vi "ScanCtrl_3D.vi"() -> ()   [LabVIEW 2024]
uses:
  <vilib>/Math Plots/3D Math Plots/3D Scatter/3D Scatter XCtrl/3D Scatter.xctl
  <vilib>/userDefined/High Color/IMAQdx.ctl
  <vilib>/vision/Image Controls.llb/IMAQ Image.ctl
  SubVI/GRBL/Status.ctl
  <vilib>/event_ctls.llb/usereventprio.ctl
  <vilib>/vision/driver/IMAQdx.llb/IMAQdx Buffer Number Mode.ctl
  <vilib>/Math Plots/3D Math Plots/3D Scatter/3D Scatter Datatype/Public/Plot Helper (Vector).vi
  <vilib>/Instr/_visa.llb/VISA Configure Serial Port (Instr).vi
  <vilib>/ErrorRing/Error Ring.xnode
  SubVI/GRBL/GRBL 1.1.lvlib
  <userlib>/_OpenG.lib/time/time.llb/openg_time.lvlib
  <vilib>/Math Plots/3D Math Plots/3D Scatter/3D Scatter Datatype/3D Scatter Datatype.lvclass
  <vilib>/vision/driver/NI_Vision_Acquisition_Software.lvlib
panel:
  in  "AbortScan":bool
  out "Estimated surface\n scan time (s)":dbl
  in  "3DProfileScan":bool
  in  "Pre Scan Speed\n(mm/min)":sgl=3000.0
  in  "Y Pixel Size(mm)":dbl=1.0
  in  "Y distance(mm)":dbl=10.0
  in  "X distance (mm)":dbl=10.0
  out "LocationPollingStart":u32
  out "error out":errorcluster
  in  "Save Button":bool
  out "Sys Status":T1
  out "dt polling (ms)":dbl
  out "X encoder count":dbl format="%.2f"
  out "Z Distance(mm)":dbl
  out "X (mm)":dbl
  in  "Range Finder COM":refnum<visa-resource-name>="COM7"
  in  "Stage COM port":refnum<visa-resource-name>="COM6"
  in  "ParseLocationData":bool
  in  "Upper Z limite(mm)":dbl=15.0
  in  "Remove Z outlier":bool
  in  "Probe Radius(2mm)":dbl=2.0 format="%#_13g"
  in  "Interpolate Scan":bool
  in  "FollowScanGridSize(mm)":dbl=0.5 format="%#_13g"
  in  "Calc follow scan":bool
  in  "Follow Z offset(mm)":dbl=3.0
  out "3D Profile":refnum<class "3D Plot Datatype.lvclass">[](xcontrol)
  in  "Follow Speed (mm/min)":sgl=1500.0
  in  "Follow Scan":bool
  in  "Plot 3D":bool
  in  "Tab Control":T2(tab)
  out "Scan Origin MPos":cluster{"X":sgl, "Y":sgl, "Z":sgl}
  in  "Set Origin":bool
  in  "Jog Step Size(mm)":dbl=5.0
  in  "Z--":bool
  in  "Z++":bool
  in  "Y--":bool
  in  "Y++":bool
  in  "X--":bool
  in  "X++":bool
  in  "Hault":bool
  in  "Home":bool
  in  "GoToZero":bool
  out "Current Machine Pos":cluster{"X":sgl, "Y":sgl, "Z":sgl}
  in  "Poll grbl position?":bool
  out "Stage Home MPos":cluster{"X":sgl, "Y":sgl, "Z":sgl}
  in  "Stop":bool
  in  "Start":bool
  in  "AccuRangeLoopStopFlag":bool
  out "read buffer":string
  out "Y Graph":dbl[](graph)
  out "X Graph":dbl[](graph)
  out "Z Graph":dbl[](graph)
  in  "X-Axis configuration":T3={"Travel resolution\t(step/mm)"=160.0, "Maximum rate\t(mm/min)"=6000, "Acceleration\t(mm/sec^2)"=1000, "Maximum travel\t(mm)"=100}
  in  "Y-Axis configuration":T3={"Travel resolution\t(step/mm)"=160.0, "Maximum rate\t(mm/min)"=2000, "Acceleration\t(mm/sec^2)"=250, "Maximum travel\t(mm)"=150}
  in  "Z-Axis configuration":T3={"Travel resolution\t(step/mm)"=160.0, "Maximum rate\t(mm/min)"=2000, "Acceleration\t(mm/sec^2)"=250, "Maximum travel\t(mm)"=70}
  out "Current Config":string="$0=10\r\n$1=255\r\n$2=0\r\n$3=0\r\n$4=0\r\n$5=1\r\n$6=0\r\n$10=1\r\n$11=0.010\r\n$12=1000.000\r\n$13=0\r\n$20=1\r\n$21=0\r\n$22=1\r\n$23=0\r\n$24=5.000\r\n$25=3000.000\r\n$26=25\r\n$27=2.000\r\n$30=12000\r\n$31=4000\r\n$32=0\r\n$100=13.333\r\n$101=13.333\r\n$102=98.000\r\n$110=50000.000\r\n$111=50000.000\r\n$112=1800.000\r\n$120=250.000\r\n$121=250.000\r\n$122=50.000\r\n$130=267.000\r\n$131=472.000\r\n$132=68.000\r\nok\r\nok\r\n"
  out "Version information":string="[VER:1.1f.20170324:]\r\n[OPT:VM,15,128]\r\nok\r\nok\r\n"
  in  "CamSession In":T4="cam0"
  out "New Image":T5
  in  "Preview":bool
  out "Image":T5(plugin-control)
  out "PPIX intensity trace":dbl(graph)
  in  "FollowScan":bool
  out "CH1":refnum<class "3D Plot Datatype.lvclass">[](xcontrol)
  out "AbortFlag":bool
  out "3D scan":errorcluster
  in  "Quit":bool
  # "3D Profile Scan Setting"
  # "Current Position"
  # "Please wait 5s between start and stop"
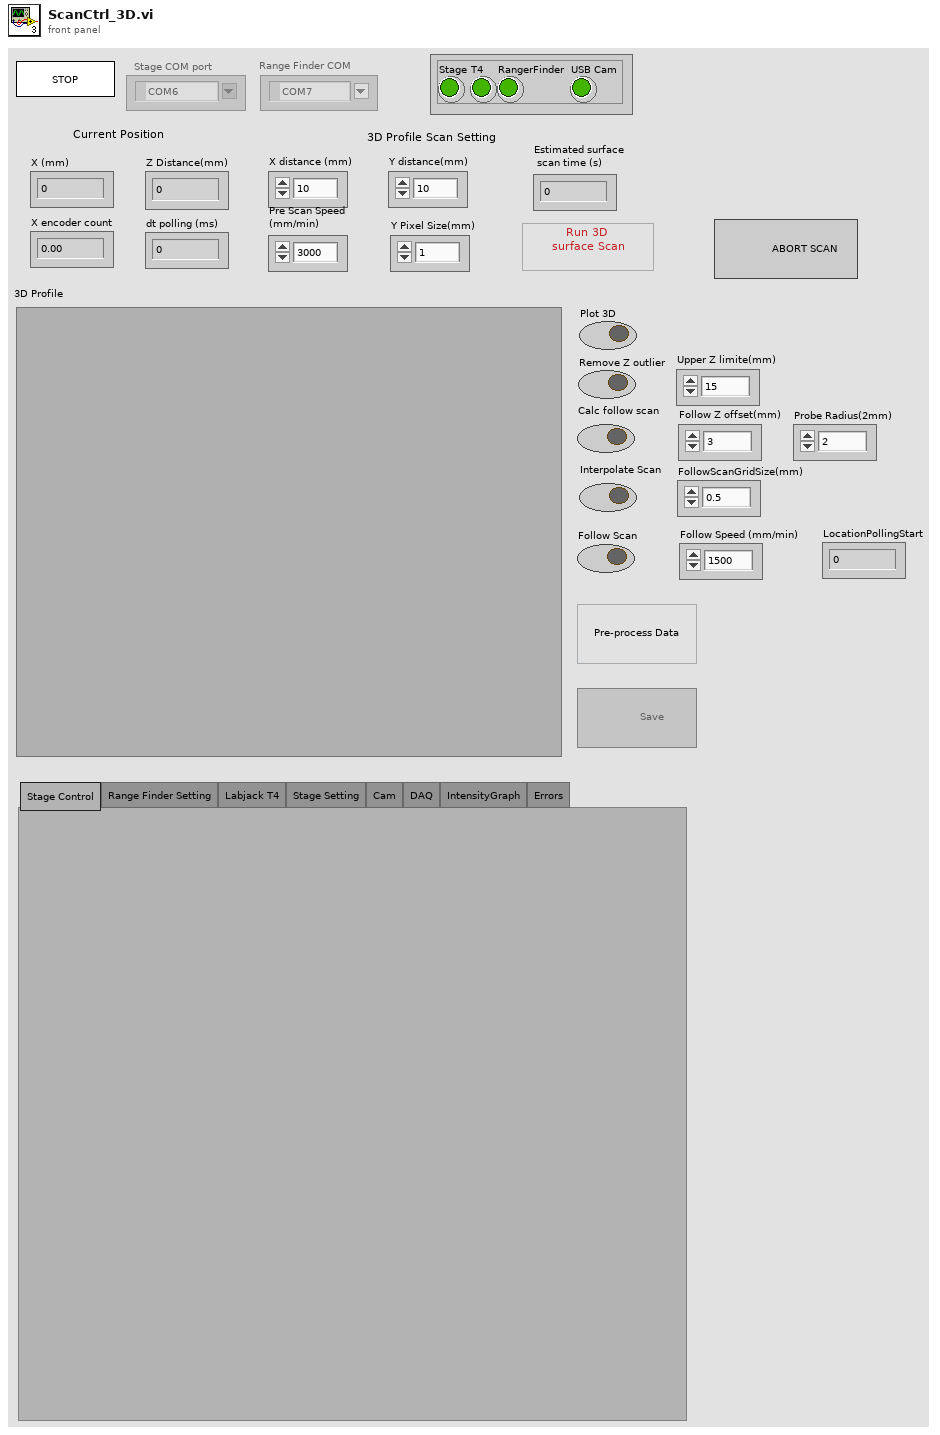
[diagram p1: front panel]
types:
  T1 = cluster{"Stage":bool, "T4":bool, "RangerFinder":bool, "USB Cam":bool}
  T2 = enum32{"Stage Control", "Range Finder Setting", "Labjack T4", "Stage Setting", "Cam", "DAQ", "IntensityGraph", "Errors"}
  T3 = cluster{"Travel resolution\t(step/mm)":sgl, "Maximum rate\t(mm/min)":u32, "Acceleration\t(mm/sec^2)":u32, "Maximum travel\t(mm)":u32}
  T4 = typedef "IMAQdx.ctl" = refnum<k21>
  T5 = typedef "IMAQ Image.ctl" = refnum<image>
  T6 = enum8{"Enabled", "Disabled", "Disabled and Grayed Out"}
  T7 = typedef "NI_Vision_Acquisition_Software.lvlib/IMAQdx Buffer Number Mode.ctl" = enum32{"Next", "Last", "Buffer Number", "Every", "Last New"}
  T8 = typedef "usereventprio.ctl" = enum32{"high priority", "normal priority"}
  T9 = typedef "GRBL 1.1.lvlib/Status.ctl" = enum16{"", "Alarm", "Idle", "Run", "Home"}
  T10 = enum32{"Invalid", "Standard", "Closed", "Hidden", "Minimized", "Maximized"}
  T11 = enum32{"invalid app kind", "Development System", "Run Time System", "Student Edition", "Embedded LabVIEW", "Evaluation", "Custom"}
  T12 = enum16{"open", "open or create", "create or replace", "create", "open (read-only)"}
  T13 = cluster{"Invert enable pin":bool, "Invert limit pin":bool, "Invert probe pin":bool}
  T14 = cluster{"Reverse X":bool, "Reverse Y":bool, "Reverse Z":bool}
  T15 = cluster{"Core":cluster{"Current VI Reference":refnum<vi>, "Close Panel on Exit?":bool}, "Sys Status":cluster{"Stage":bool, "T4":bool, "RangerFinder":bool, "USB Cam":bool}, "StageCOM":refnum<visa-resource-name>, "RangeCOM":refnum<visa-resource-name>, "StepSize":dbl, "ScanOrigin":cluster{"X":sgl, "Y":sgl, "Z":sgl}, "HomeMposOrigin":cluster{"X":sgl, "Y":sgl, "Z":sgl}, "Tic":i32, "IMAQ":T5, "USBCam":T4, "3DProfile":cluster{"x(mm)":dbl, "y(mm)":dbl, "z(mm)":dbl}[], "Raw3DProfile":cluster{"x(mm)":dbl, "y(mm)":dbl, "z(mm)":dbl}[], "FollowScanZOffset(mm)":dbl, "YPixelSize(mm)":dbl, "FollowScanWInter":cluster{"x(mm)":dbl, "y(mm)":dbl, "z(mm)":dbl}[], "BG(V)":dbl, "StageHomed?":bool, "3DProfileToPlot":cluster{"x(mm)":dbl, "y(mm)":dbl, "z(mm)":dbl}[], "FollowScan":cluster{"x(mm)":dbl, "y(mm)":dbl, "z(mm)":dbl}[], "SaveFilePath":path, "Raw3DProfileNoY":cluster{"x(mm)":dbl, "y(mm)":dbl, "z(mm)":dbl}[], "tdms file":refnum<k34>, "FiberOffset":cluster{"x":dbl, "y":dbl}, "RawFollowScanData":cluster{"Time(ms)":dbl, "x":dbl}[], "PPIXProcessedImg":cluster{"x":dbl[], "y":dbl[], "Time(ms)":dbl[]}, "ProbeRadius(mm)":dbl, "FollowGridSize(mm)":dbl}
  T16 = cluster{"remote start event":refnum<user-event>, "remote stop event":refnum<user-event>}
  T17 = cluster{"Current VI Reference":refnum<vi>, "Close Panel on Exit?":bool}
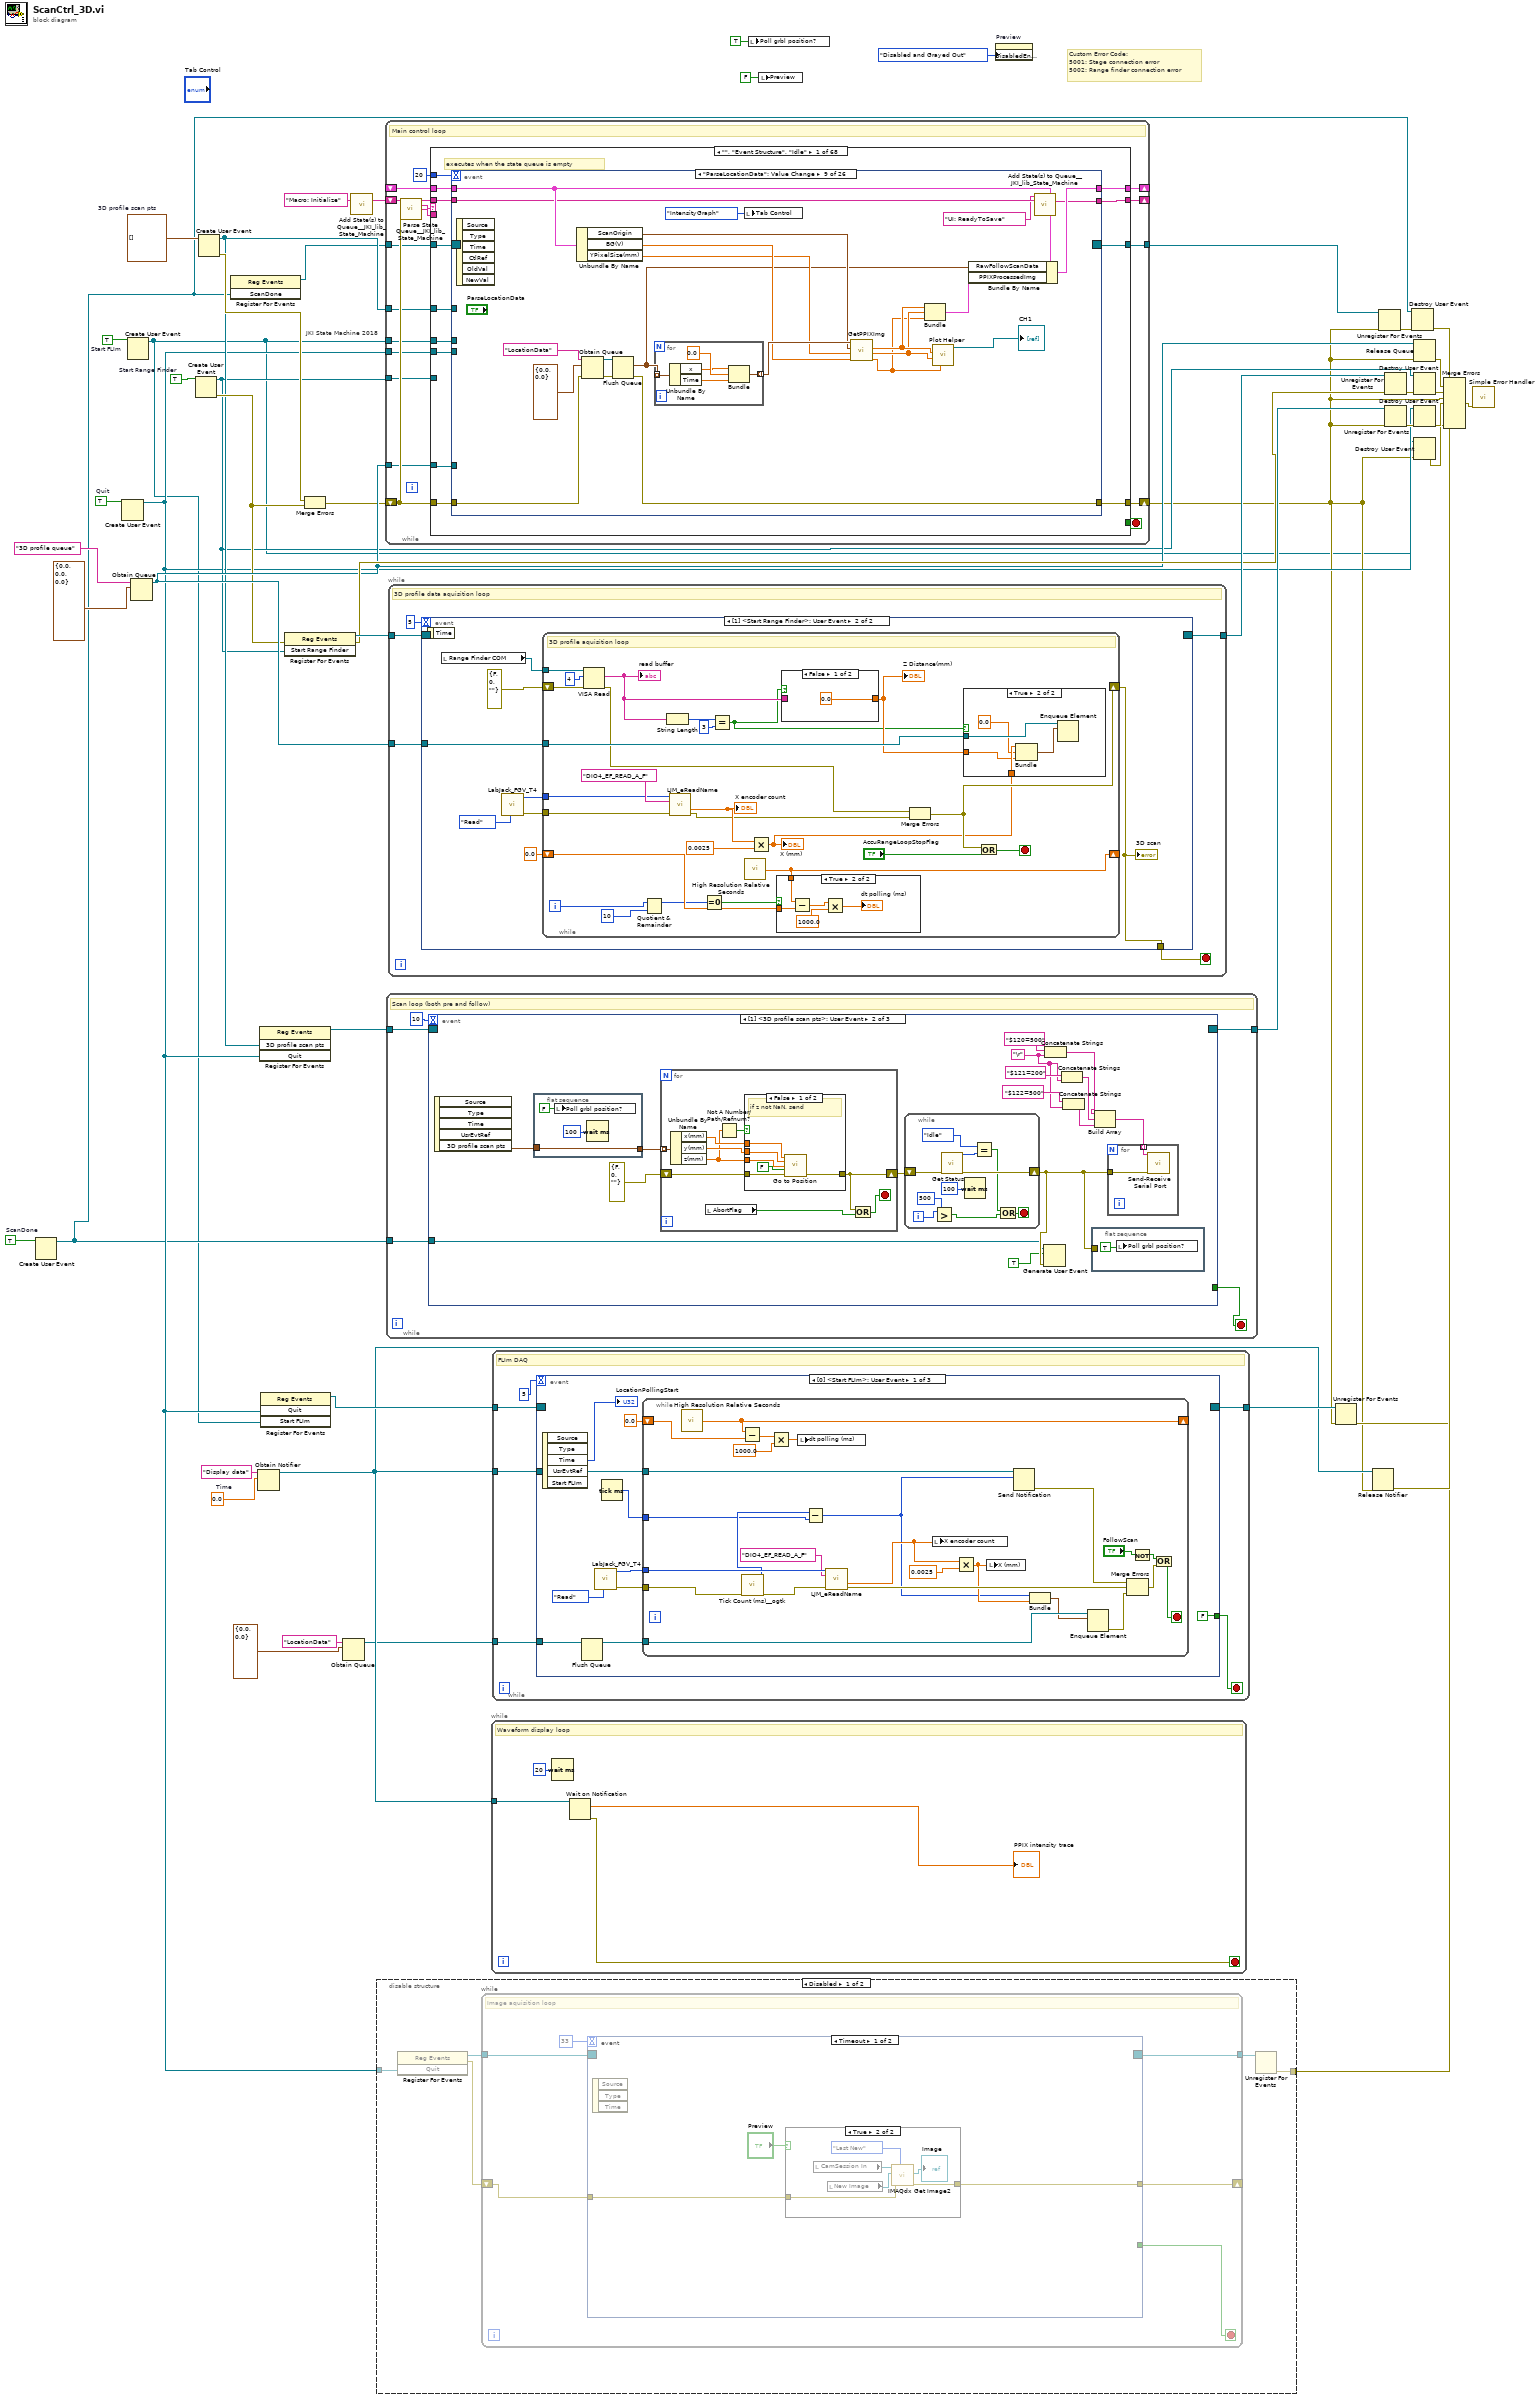
[diagram p0: block diagram]
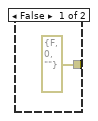
[diagram p2: hidden frame]
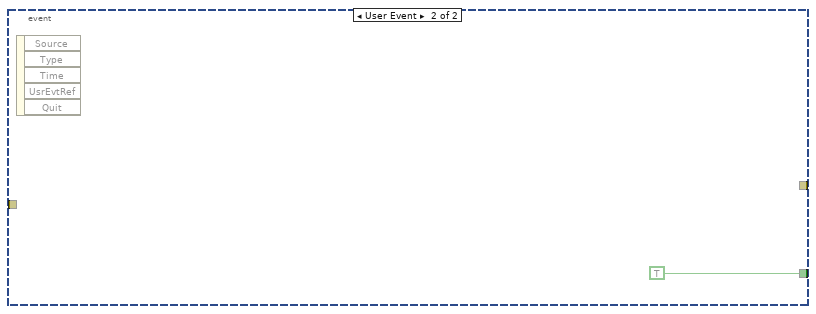
[diagram p3: hidden frame]
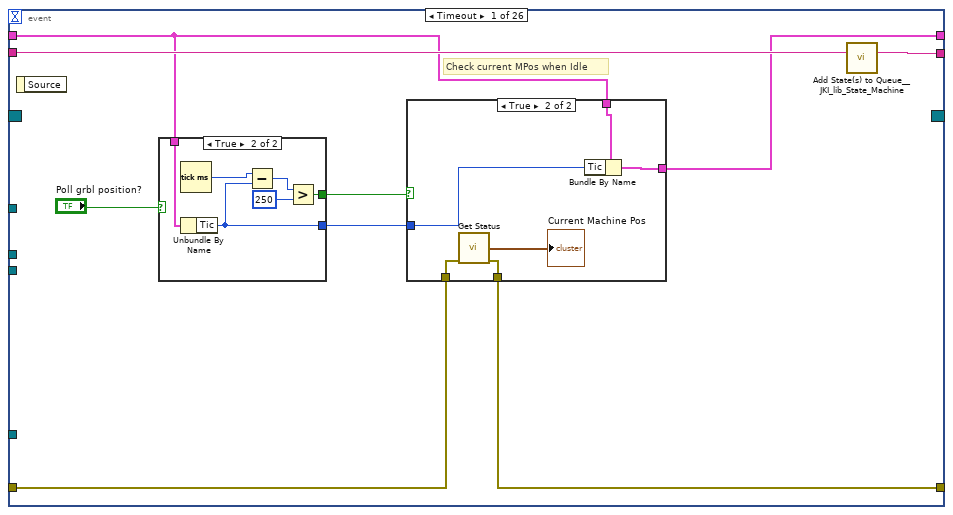
[diagram p5: hidden frame]
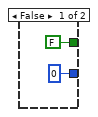
[diagram p6: hidden frame]
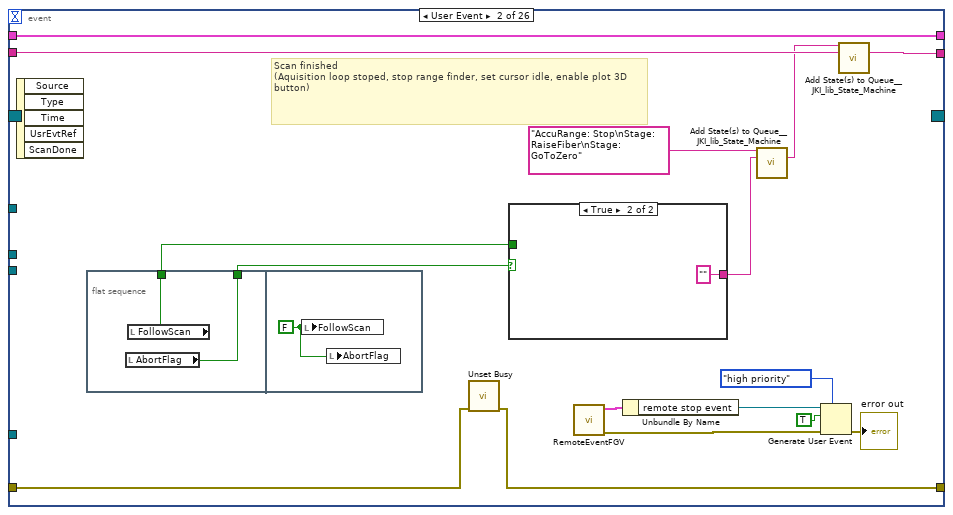
[diagram p8: hidden frame]
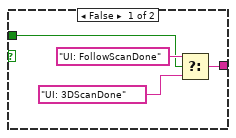
[diagram p9: hidden frame]
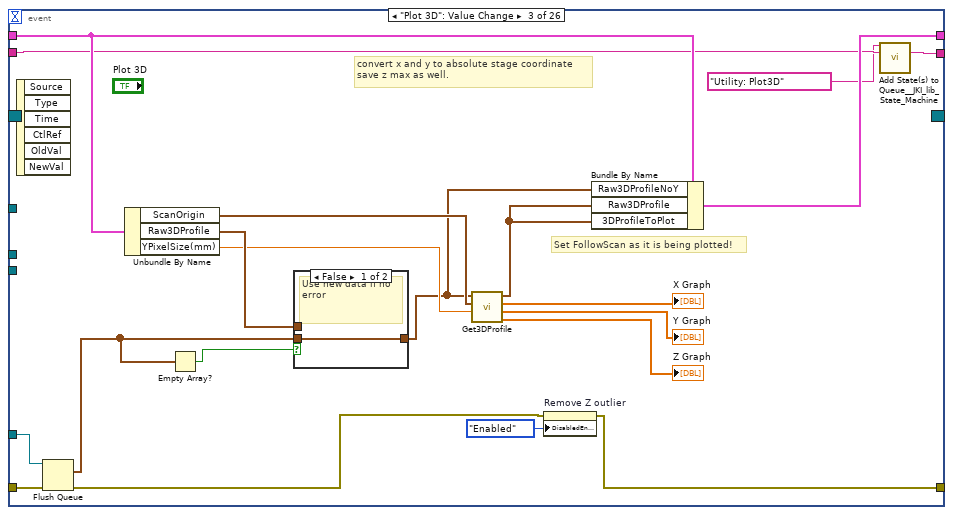
[diagram p10: hidden frame]
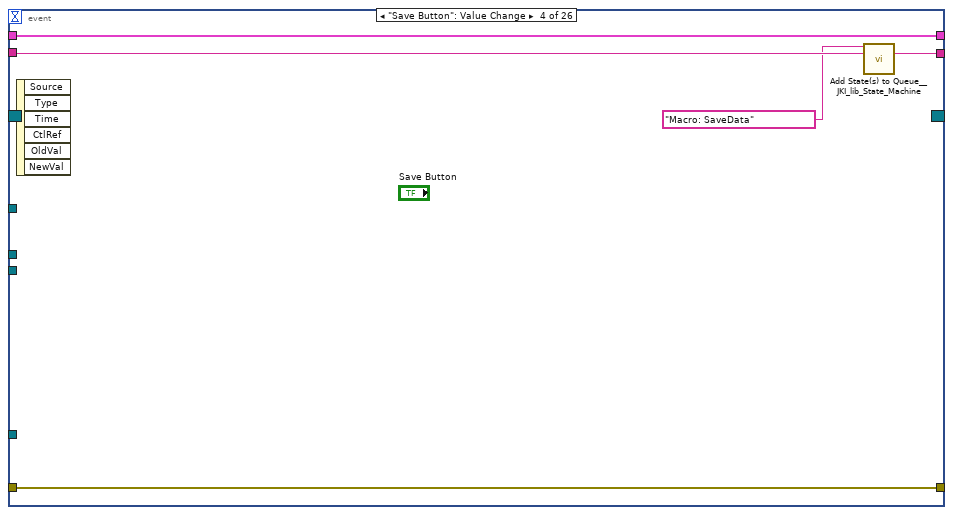
[diagram p12: hidden frame]
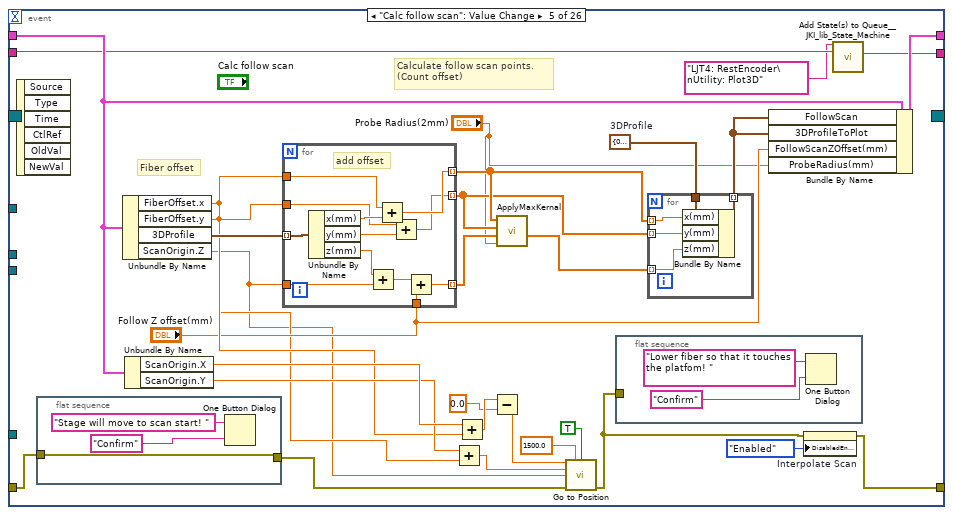
[diagram p13: hidden frame]
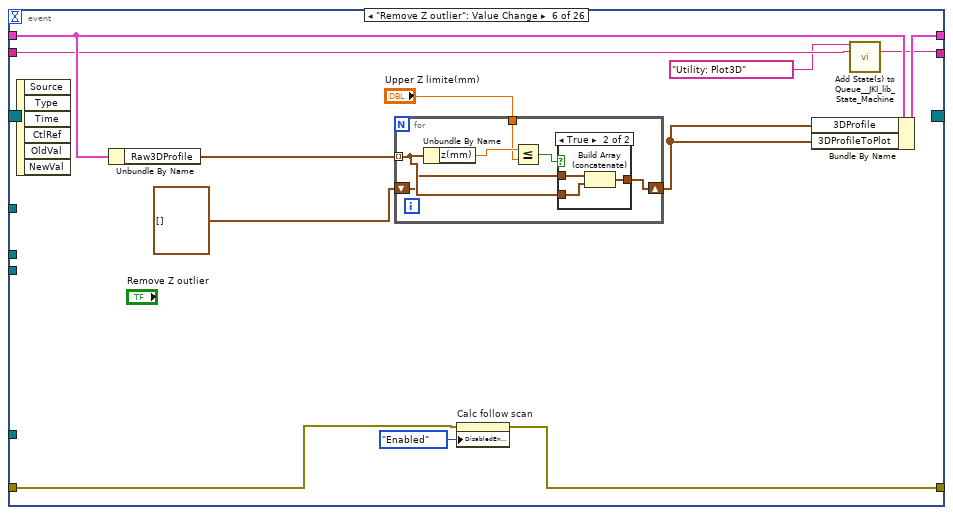
[diagram p14: hidden frame]
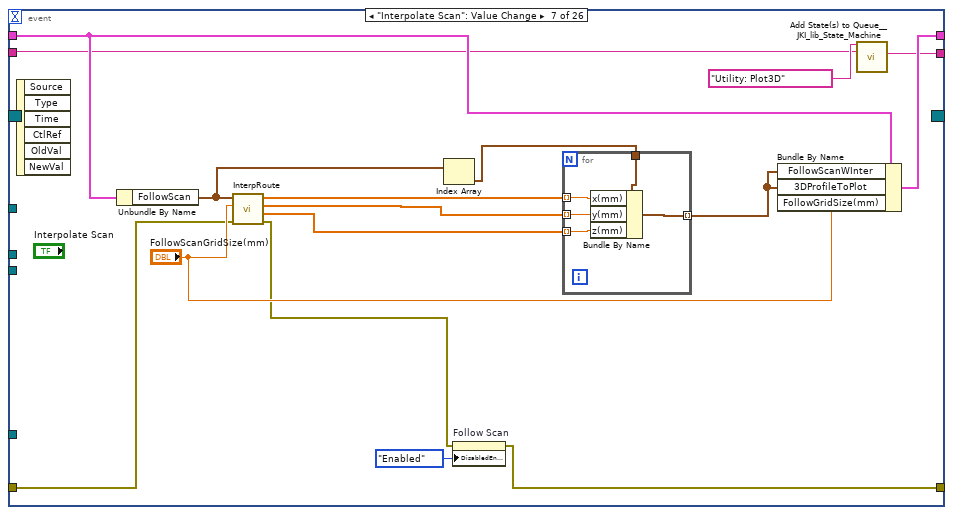
[diagram p16: hidden frame]
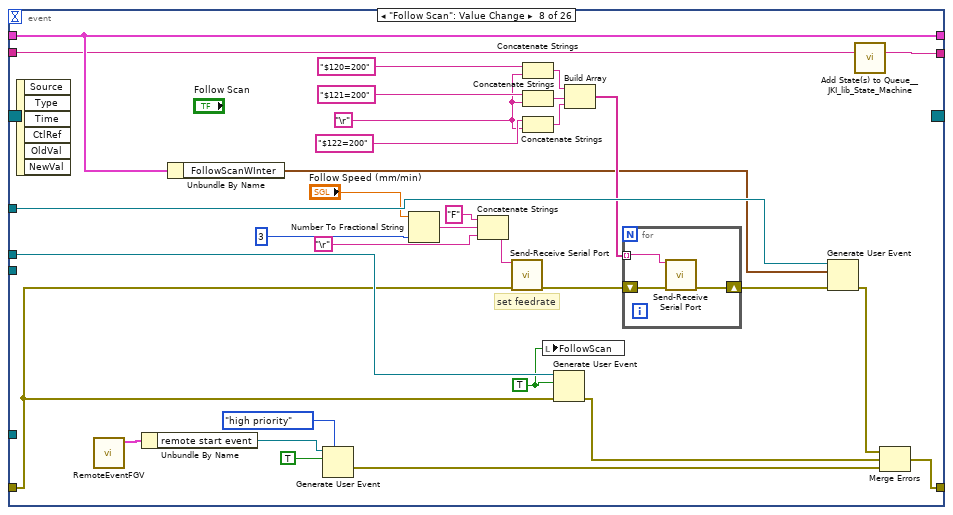
[diagram p17: hidden frame]
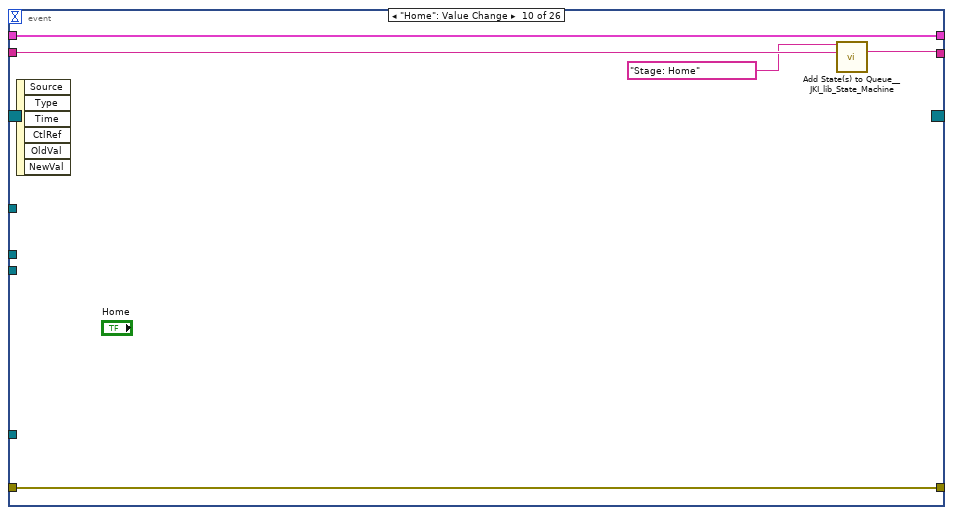
[diagram p18: hidden frame]
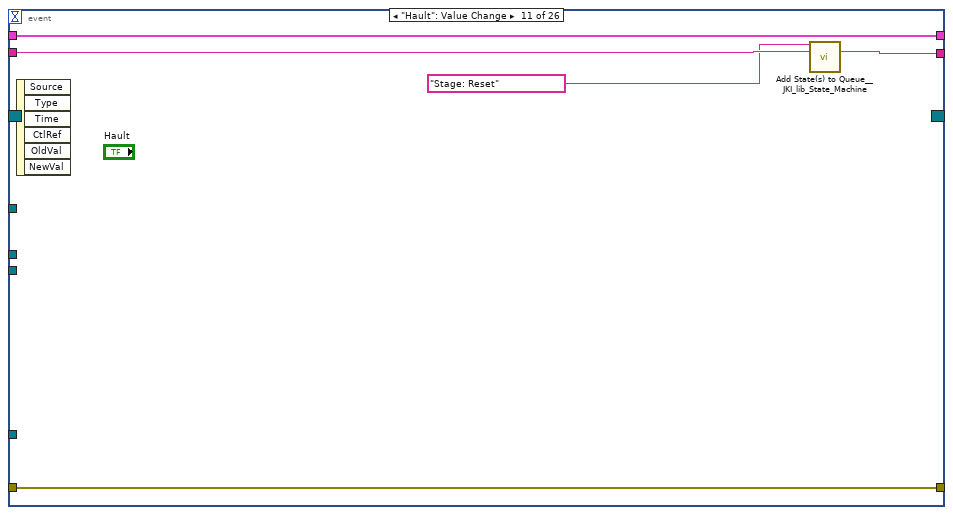
[diagram p19: hidden frame]
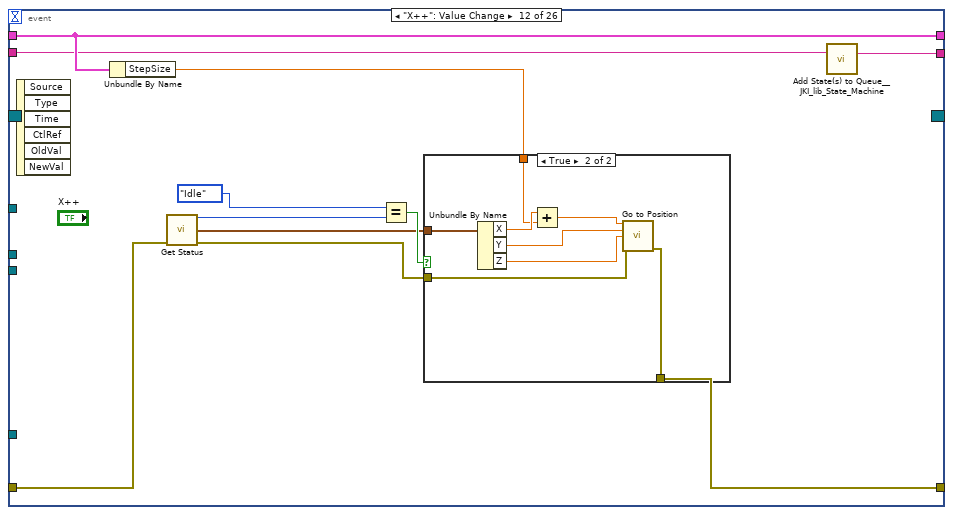
[diagram p20: hidden frame]
diagram:
  w3 = 0.0  # Time
  w12 = TRUE  # ScanDone
  w15 = TRUE  # Start FLIm
  w27 = TRUE  # Quit
  w28 = cluster{"x(mm)":dbl, "y(mm)":dbl, "z(mm)":dbl}[] []  # 3D profile scan pts
  w47 = TRUE  # Start Range Finder
  # "Custom Error Code:\n5001: Stage connection error\n5002: Range finder connection error"
  n1 = Create User Event(user event datatype=w12) -> (user event=w8:refnum<user-event>)  [unwired: 1 in, 1 out]
  n2 = Create User Event(user event datatype=w27) -> (user event=w19:refnum<user-event>)  [unwired: 1 in, 1 out]
  n3 = Create User Event(user event datatype=w15) -> (user event=w1:refnum<user-event>)  [unwired: 1 in, 1 out]
  n4 = Obtain Queue(name (unnamed)="3D profile queue", element data type=cluster{"x(mm)":dbl, "y(mm)":dbl, "z(mm)":dbl} {"x(mm)"=0.0, "y(mm)"=0.0, "z(mm)"=0.0}) -> (queue out=w38:refnum<queue>)  [unwired: 3 in, 2 out]
  n5 = Create User Event(user event datatype=w47) -> (user event=w29:refnum<user-event>, error out=w34:errorcluster)  [unwired: 1 in]
  n6 = Create User Event(user event datatype=w28) -> (user event=w31:refnum<user-event>, error out=w32:errorcluster)  [unwired: 1 in]
  n7 = register-events(w8) -> (reference out=w11:refnum<event-registration>)  [unwired: 2 in, 1 out]
  n8 = Obtain Notifier(name (unnamed)="Display data", notification data type=w3) -> (notifier out=w13:refnum<notifier>)  [unwired: 2 in, 2 out]
  n9 = register-events(w31, w19) -> (reference out=w26:refnum<event-registration>)  [unwired: 2 in, 1 out]
  n10 = register-events(w19, w1) -> (reference out=w22:refnum<event-registration>)  [unwired: 2 in, 1 out]
  n11 = register-events(error in=w34, w29) -> (reference out=w46:refnum<event-registration>, error out=w43:errorcluster)  [unwired: 1 in]
  n12 = Merge Errors(w32, w34) -> (w35:errorcluster)
  n13 = Obtain Queue(name (unnamed)="LocationData", element data type=cluster{"Time":dbl, "x":dbl} {"Time"=0.0, "x"=0.0}) -> (queue out=w4:refnum<queue>)  [unwired: 3 in, 2 out]
  n14 = call <vilib>:"Add State(s) to Queue__JKI_lib_State_Machine.vi"("State(s) in (\"\")"="Macro: Initialize") -> ("States Out"=w49:string)  [unwired: 14 in]
  n15 = disable-structure shown="Disabled" {
    disable-tunnel: w19 -> [w54 _]
    disable-tunnel: [w53 _] -> w18
    frame Disabled {
      n16 = register-events(w54) -> (reference out=w52:refnum<event-registration>, error out=w51:errorcluster)  [unwired: 2 in]
      n17 = while {
        shift-right: [w59] -> _
        shift-left: w51 -> [w58]
        tunnel: w52 -> [w57]
        tunnel: [w55] -> w50
        stop <- w56 stop-if-true
        # "Image aquisition loop"
        n18 = event shown="[0] Timeout" {
          selector: w57 -> [_ _]
          dyn-events: [_ _] -> w55
          timeout: u32 33 ("milliseconds to wait") -> [_ _]
          tunnel: [w62 _] -> w59
          tunnel: w58 -> [w61 _]
          tunnel: [_ TRUE] -> w56
          event Timeout {
            n19 = event-data() -> ()  [unwired: 1 in, 3 out]
            n20 = case shown="True" "Preview" {
              tunnel: [errorcluster {"status"=FALSE, "code"=0, "source"=""} ("error out") w66] -> w62
              tunnel: w61 -> [_ w65]
              frame False {
              }
              frame True {
                n21 = local read "CamSession In"() -> (w68:T4)
                n22 = local read "New Image"() -> (w69:T5)
                n23 = call <vilib>:"IMAQdx Get Image2.vi"("Buffer Number Mode (Next)"=IMAQdx_Buffer_Number_Mode."Last New", "error in"=w65, "Image In"=w69, "Session In"=w68) -> ("error out"=w66:errorcluster, "Image Out"=→"Image":T5)  [unwired: 4 in, 2 out]
              }
            }
          }
          event User Event {
            n24 = event-data() -> ()  [unwired: 1 in, 5 out]
          }
        }
      }
      n25 = Unregister For Events(event registration refnum=w50) -> (error out=w53:errorcluster)  [unwired: 1 in]
    }
    frame Enabled {
    }
  }
  n26 = while "JKI State Machine 2018" {
    shift-right: [w84] -> _
    shift-left: _ -> [w72]
    shift-right: [w87] -> w9
    shift-left: w35 -> [w82]
    shift-right: [w86] -> _
    shift-left: w49 -> [w80]
    tunnel: w29 -> [w81]
    tunnel: w38 -> [w79]
    tunnel: w31 -> [w78]
    tunnel: w19 -> [w77]
    tunnel: w1 -> [w76]
    tunnel: w11 -> [w74]
    tunnel: [w73] -> w10
    stop <- w85 stop-if-true
    # "Main control loop"
    n27 = call <vilib>:"Parse State Queue__JKI_lib_State_Machine.vi"("State Queue"=w80, "Error In (no error)"=w82) -> ("Remaining States"=w89:string, "Current State"=w75:string, "Arguments"=w88:string)  [unwired: 11 in]
    n28 = case shown="\"\", \"Event Structure\", \"Idle\"" w75 {
      selector: w75 -> [_ _ _ _ _ _ w594 _ _ _ _ _ _ _ _ _ _ _ _ _ _ _ _ _ _ _ _ _ _ _ _ _ _ _ _ _ _ _ _ _ _ _ _ _ _ _ _ _ _ _ _ _ _ _ _ _ _ _ _ _ _ _ _ _ _ _ _ _]
      tunnel: w89 -> [w102 w563 w564 w575 w587 w592 w598 w618 w625 w634 w639 w671 w678 w685 w708 w721 w749 w771 w812 w840 w872 w889 w896 w912 w923 w929 w936 w942 w949 w955 w960 w968 w975 w982 w994 w1064 w1076 w1094 w1125 w1136 w1159 w1224 w1244 w1252 w1264 w1280 w1312 w1336 w1349 w1374 w1389 w1399 w1409 w1420 w1425 w1437 w1447 w1465 w1473 w1488 w1505 w1520 w1530 w1545 w1554 w1559 w1564 w1569]
      tunnel: w88 -> [_ _ _ _ _ _ _ _ _ _ _ _ _ _ _ _ _ _ _ _ _ _ _ _ _ _ _ _ _ _ _ _ _ w977 w988 _ _ _ _ _ _ _ w1239 _ _ _ _ _ _ _ _ _ _ w1416 _ _ _ _ _ _ _ _ _ _ _ _ _ _]
      tunnel: w72 -> [w100 w560 w567 w572 w584 w589 w596 w611 w622 w632 w636 _ w674 w680 w702 w718 w746 w768 w809 w837 w869 w886 w893 w903 w920 w926 w933 w939 w946 w952 w957 w965 w973 w980 w990 w1061 w1066 w1092 w1106 w1132 w1153 w1222 w1242 w1246 w1261 w1274 w1310 w1333 w1347 w1367 w1386 w1397 w1405 w1417 w1422 w1432 w1445 w1463 w1467 w1485 w1499 w1513 w1523 w1542 w1550 w1556 w1561 w1566]
      tunnel: [w99 w561 w568 w573 w585 w590 w600 w615 errorcluster {"status"=FALSE, "code"=0, "source"=""} ("error out") w628 w637 w668 w676 w681 w704 w711 w722 w756 w776 w817 w848 w880 w891 w898 w921 w927 w934 w940 w947 w953 w958 w966 w972 w978 w991 w1062 w1070 w1091 w1100 w1134 w1156 w1212 w1241 w1250 w1262 w1265 w1294 w1328 w1343 w1371 w1387 w1392 w1407 w1418 w1423 w1434 w1439 w1450 w1471 w1486 w1498 w1516 w1527 w1543 w1552 w1557 w1562 w1567] -> w87
      tunnel: w82 -> [w98 w561 w568 w573 w585 w590 w599 w615 w621 w627 w637 w668 w676 w682 w703 w716 w729 w755 w797 w825 w862 w882 w890 w897 w921 w927 w934 w940 w947 w953 w958 w966 w972 w979 w992 w1062 w1074 w1090 w1105 w1130 w1157 w1211 w1240 w1249 w1262 w1276 w1295 w1326 w1345 w1370 w1387 w1391 w1407 w1418 w1423 w1430 w1438 w1449 w1470 w1486 w1500 w1515 w1526 w1543 w1552 w1557 w1562 w1567]
      tunnel: [w101 w562 w569 w574 w586 w591 w597 w617 w624 w633 w638 w670 w677 w684 w707 w720 w748 w770 w811 w839 w871 w888 w895 w911 w922 w928 w935 w941 w948 w954 w959 w967 w974 w981 w993 w1063 w1075 w1093 w1124 w1135 w1158 w1223 w1243 w1251 w1263 w1279 w1311 w1335 w1348 w1373 w1388 w1398 w1408 w1419 w1424 w1436 w1446 w1464 w1472 w1487 w1504 w1519 w1529 w1544 w1553 w1558 w1563 w1568] -> w86
      tunnel: [_ _ _ _ _ _ _ _ _ TRUE _ _ _ _ _ _ _ _ _ _ _ _ _ _ _ _ _ _ _ _ _ _ _ _ _ _ _ _ _ _ _ _ _ _ _ _ _ _ _ _ _ _ _ _ _ _ _ _ _ _ _ _ _ _ _ _ _ _] -> w85
      tunnel: [w97 w560 w567 w572 w584 w589 w596 w616 w622 w632 w636 w669 w675 w680 w701 w718 w746 w768 w809 w837 w869 w886 w893 w902 w920 w926 w933 w939 w946 w952 w957 w965 w973 w980 w990 w1061 w1073 w1092 w1106 w1133 w1155 w1222 w1242 w1247 w1261 w1273 w1310 w1333 w1347 w1368 w1386 w1397 w1405 w1417 w1422 w1433 w1445 w1463 w1468 w1485 w1496 w1513 w1524 w1542 w1550 w1556 w1561 w1566] -> w84
      tunnel: 20 ("Timeout") -> [w96 _ _ _ _ _ _ _ _ _ _ _ _ _ _ _ _ _ _ _ _ _ _ _ _ _ _ _ _ _ _ _ _ _ _ _ _ _ _ _ _ _ _ _ _ _ _ _ _ _ _ _ _ _ _ _ _ _ _ _ _ _ _ _ _ _ _ _]
      tunnel: w81 -> [_ _ _ _ _ _ _ _ _ _ _ _ _ _ _ _ _ _ _ _ _ _ _ _ _ _ _ _ _ _ _ _ _ _ _ _ _ _ _ _ _ _ _ _ _ _ _ w1332 _ _ _ _ _ _ _ _ _ _ _ _ _ _ _ _ _ _ _ _]
      tunnel: w79 -> [w95 _ _ _ _ _ _ _ _ _ _ _ _ _ _ _ _ _ _ _ _ _ _ _ _ _ _ _ _ _ _ _ _ _ _ _ _ _ _ _ _ _ _ _ _ _ _ _ _ _ _ _ _ _ _ _ _ _ _ _ _ _ _ _ _ _ _ _]
      tunnel: w78 -> [w94 _ _ _ _ _ _ _ _ _ _ _ _ _ _ _ _ _ _ _ _ _ _ _ _ _ _ _ _ _ _ _ _ _ _ _ _ _ _ _ _ _ _ _ _ _ _ _ _ _ _ _ _ _ _ _ _ _ _ _ _ _ _ _ _ _ _ _]
      tunnel: w77 -> [w93 _ _ _ _ _ _ _ _ w629 _ _ _ _ _ _ _ _ _ _ _ _ _ _ _ _ _ _ _ _ _ _ _ _ _ _ _ _ _ _ _ _ _ _ _ _ _ _ _ _ _ _ _ _ _ _ _ _ _ _ _ _ _ _ _ _ _ _]
      tunnel: w76 -> [w92 _ _ _ _ _ _ _ _ _ _ _ _ _ _ _ _ _ _ _ _ _ _ _ _ _ _ _ _ _ _ _ _ _ _ _ _ _ _ _ _ _ _ _ _ _ _ _ _ _ _ _ _ _ _ _ _ _ _ _ _ _ _ _ _ _ _ _]
      tunnel: w74 -> [w91 w559 w565 w571 w576 w588 w593 w605 w619 w626 w635 w651 w672 w679 w706 w719 w747 w769 w810 w838 w870 w887 w894 w910 w919 w925 w932 w938 w945 w951 w956 w964 w971 w976 w987 w1060 w1068 w1089 w1096 w1131 w1154 w1221 w1238 w1245 w1260 w1266 w1293 w1313 w1339 w1366 w1385 w1396 w1400 w1414 w1421 w1431 w1444 w1448 w1466 w1484 w1489 w1511 w1522 w1541 w1551 w1555 w1560 w1565]
      tunnel: [w90 w559 w565 w571 w576 w588 w593 w605 w619 w626 w635 w651 w672 w679 w706 w719 w747 w769 w810 w838 w870 w887 w894 w910 w919 w925 w932 w938 w945 w951 w956 w964 w971 w976 w987 w1060 w1068 w1089 w1096 w1131 w1154 w1221 w1238 w1245 w1260 w1266 w1293 w1313 w1339 w1366 w1385 w1396 w1400 w1414 w1421 w1431 w1444 w1448 w1466 w1484 w1489 w1511 w1522 w1541 w1551 w1555 w1560 w1565] -> w73
      frame "", "Event Structure", "Idle" {
        # "executes when the state queue is empty"
        n29 = event shown="[8] \"ParseLocationData\": Value Change" {
          selector: w91 -> [_ _ _ _ _ _ _ _ _ _ _ _ _ _ _ _ _ _ _ _ _ _ _ _ _ _]
          dyn-events: [_ _ _ _ _ _ _ _ _ _ _ _ _ _ _ _ _ _ _ _ _ _ _ _ _ _] -> w90
          timeout: w96 -> [_ _ _ _ _ _ _ _ _ _ _ _ _ _ _ _ _ _ _ _ _ _ _ _ _ _]
          tunnel: w102 -> [w111 w141 w165 w176 w197 w238 w259 w285 w311 w338 w344 w354 w375 w389 w401 w422 w443 w463 w478 w508 w520 w535 w542 w546 w551 w558]
          tunnel: [w110 w142 w164 w177 w198 w237 w258 w286 w310 w339 w343 w355 w376 w390 w402 w423 w444 w463 w477 w508 w521 w535 w541 w545 w550 w557] -> w101
          tunnel: w100 -> [w105 w143 w168 w175 w206 w240 w266 w305 w317 w340 w345 w356 w377 w392 w403 w424 w445 w466 w473 w510 w522 w537 w540 w547 w552 w555]
          tunnel: [w109 w131 w154 w178 w200 w233 w261 w281 w325 w337 w341 w347 w368 w391 w394 w415 w436 w456 w470 w511 w513 w533 w538 w543 w548 w556] -> w99
          tunnel: w98 -> [w108 w133 w170 w178 w195 w232 w254 w283 w327 w337 w341 w346 w367 w391 w393 w414 w435 w461 w475 w511 w512 w533 w538 w543 w548 w556]
          tunnel: [w106 w143 w169 w175 w207 w239 w265 w305 w318 w340 w345 w356 w377 w392 w403 w424 w445 w465 w474 w510 w522 w536 w540 w547 w552 w555] -> w97
          tunnel: w95 -> [_ _ w171 _ _ _ _ _ _ _ _ _ _ _ _ _ _ _ w476 _ _ _ _ _ _ _]
          tunnel: w94 -> [_ _ _ _ _ _ _ w304 _ _ _ _ _ _ _ _ _ _ w471 _ _ _ _ _ _ _]
          tunnel: w93 -> [_ _ _ _ _ _ _ _ _ _ _ _ _ _ _ _ _ _ _ _ _ _ _ _ _ _]
          tunnel: w92 -> [_ _ _ _ _ _ _ w284 _ _ _ _ _ _ _ _ _ _ _ _ _ _ _ _ _ _]
          event Timeout {
            # "Check current MPos when Idle"
            n30 = event-data() -> ()  [unwired: 1 in, 1 out]
            n31 = case shown="True" "Poll grbl position?" {
              tunnel: [FALSE w116] -> w107
              tunnel: w105 -> [_ w115]
              tunnel: [0 ("Tic") w114] -> w104
              frame False {
              }
              frame True {
                n32 = Tick Count (ms)() -> (millisecond timer value=w119:u32)
                n33 = Unbundle By Name(w115) -> ("Tic"=w114:i32)
                n34 = Subtract(x=w119, y=w114) -> (x-y=w118:u32)
                n35 = Greater?(x=w118, y=u32 250) -> (0:w116:bool)
              }
            }
            n36 = case shown="True" w107 {
              tunnel: [w121 w127] -> w109
              tunnel: w108 -> [w121 w126]
              tunnel: w105 -> [w120 w124]
              tunnel: [w120 w123] -> w106
              tunnel: w104 -> [_ w122]
              frame False {
              }
              frame True {
                n37 = call "Get Status.vi"("error in (no error)"=w126) -> ("Current position"=→"Current Machine Pos":cluster{"X":sgl, "Y":sgl, "Z":sgl}, "error out"=w127:errorcluster)  [unwired: 10 in, 3 out]
                n38 = Bundle By Name(cluster=w124, "Tic"=w122) -> (w123:T15)
              }
            }
            n39 = call <vilib>:"Add State(s) to Queue__JKI_lib_State_Machine.vi"("State(s) in (\"\")"=w111) -> ("States Out"=w110:string)  [unwired: 14 in]
          }
          event User Event {
            # "Scan finished\n(Aquisition loop stoped, stop range finder, set cursor idle, enable plot 3D button)"
            n40 = event-data() -> ()  [unwired: 1 in, 5 out]
            n41 = flat-sequence {
              tunnel: [w150] -> w140
              tunnel: [w149] -> w128
              frame #0 {
                n42 = local read "AbortFlag"() -> (w149:bool)
                n43 = local read "FollowScan"() -> (w150:bool)
              }
              frame #1 {
                w151 = FALSE ("InScan")
                n44 = local write "FollowScan"(w151) -> ()
                n45 = local write "AbortFlag"(w151) -> ()
              }
            }
            n46 = call <vilib>:"Unset Busy.vi"("error in (no error)"=w133) -> ("error out"=w131:errorcluster)  [unwired: 10 in]
            n47 = case shown="True" w128 {
              tunnel: w140 -> [w145 _]
              tunnel: [w144 "" ("State(s) in (\"\")")] -> w138
              frame False {
                n48 = Select(t="UI: FollowScanDone", s=w145, f="UI: 3DScanDone" ("State(s) in (\"\")")) -> (s? t:f=w144:string)
              }
              frame True {
              }
            }
            n49 = call "RemoteEventFGV.vi"() -> ("Error Out"=w132:errorcluster, "Remote Event out"=w136:T16)  [unwired: 10 in]
            n50 = Unbundle By Name(w136) -> ("remote stop event"=w135:refnum<user-event>)
            n51 = call <vilib>:"Add State(s) to Queue__JKI_lib_State_Machine.vi"("State(s) in Front (\"\")"="AccuRange: Stop\nStage: RaiseFiber\nStage: GoToZero" ("State(s) in (\"\")"), "State(s) in (\"\")"=w138) -> ("States Out"=w137:string)  [unwired: 13 in]
            n52 = Generate User Event(priority (normal)=usereventprio."high priority", user event=w135, event data cluster=TRUE ("event data"), error in=w132) -> (error out=→"error out":errorcluster)  [unwired: 1 out]
            n53 = call <vilib>:"Add State(s) to Queue__JKI_lib_State_Machine.vi"("State(s) in Front (\"\")"=w137, "State(s) in (\"\")"=w141) -> ("States Out"=w142:string)  [unwired: 13 in]
          }
          event "Plot 3D": Value Change {
            # "Set FollowScan as it is being plotted!"
            # "convert x and y to absolute stage coordinate\nsave z max as well."
            n54 = event-data() -> ()  [unwired: 1 in, 6 out]
            n55 = Flush Queue(queue=w171, error in (no error)=w170) -> (remaining elements=w159:cluster{"x(mm)":dbl, "y(mm)":dbl, "z(mm)":dbl}[], error out=w155:errorcluster)  [unwired: 1 out]
            n56 = Unbundle By Name(w168) -> ("ScanOrigin"=w167:cluster{"X":sgl, "Y":sgl, "Z":sgl}, "Raw3DProfile"=w162:cluster{"x(mm)":dbl, "y(mm)":dbl, "z(mm)":dbl}[], "YPixelSize(mm)"=w161:dbl)
            n57 = Empty Array?(array=w159) -> (empty?=w158:bool)
            n58 = case shown="False" w158 {
              tunnel: w159 -> [w172 _]
              tunnel: [w172 w173] -> w152
              tunnel: w162 -> [_ w173]
              frame False {
                # "Use new data if no error"
              }
              frame True {
                # "Use old data if error"
              }
            }
            n59 = call "Get3DProfile.vi"("dy"=w161, "Origin"=w167, "remaining elements"=w152) -> ("Z"=→"Z Graph":dbl[], "Y"=→"Y Graph":dbl[], "X"=→"X Graph":dbl[], "3D Profile"=w156:cluster{"x(mm)":dbl, "y(mm)":dbl, "z(mm)":dbl}[])  [unwired: 5 in]
            n60 = property on="Remove Z outlier" class="Bool"(error in=w155, "DisabledEnum"=T6."Enabled" ("Disabled")) -> (error out=w154:errorcluster)  [unwired: 1 in, 1 out]
            n61 = Bundle By Name(cluster=w168, "Raw3DProfileNoY"=w152, "Raw3DProfile"=w156, "3DProfileToPlot"=w156) -> (w169:T15)
            n62 = call <vilib>:"Add State(s) to Queue__JKI_lib_State_Machine.vi"("State(s) in Front (\"\")"="Utility: Plot3D" ("State(s) in Front (\"\")"), "State(s) in (\"\")"=w165) -> ("States Out"=w164:string)  [unwired: 13 in]
          }
          event "Save Button": Value Change {
            n63 = event-data() -> ()  [unwired: 1 in, 6 out]
            n64 = call <vilib>:"Add State(s) to Queue__JKI_lib_State_Machine.vi"("State(s) in Front (\"\")"="Macro: SaveData" ("State(s) in Front (\"\")"), "State(s) in (\"\")"=w176) -> ("States Out"=w177:string)  [unwired: 13 in]
          }
          event "Calc follow scan": Value Change {
            w188 = cluster{"x(mm)":dbl, "y(mm)":dbl, "z(mm)":dbl} {"x(mm)"=0.0, "y(mm)"=0.0, "z(mm)"=0.0}  # 3DProfile
            # "Fiber offset"
            # "Calculate follow scan points.\n(Count offset)"
            n65 = event-data() -> ()  [unwired: 1 in, 6 out]
            n66 = flat-sequence {
              tunnel: w195 -> [w216]
              tunnel: [w216] -> w179
              frame #0 {
                n67 = One Button Dialog(message="Stage will move to scan start! ", button name ("OK")="Confirm") -> ()  [unwired: 1 out]
              }
            }
            n68 = Unbundle By Name(w206) -> ("FiberOffset.x"=w193:dbl, "FiberOffset.y"=w185:dbl, "3DProfile"=w208:cluster{"x(mm)":dbl, "y(mm)":dbl, "z(mm)":dbl}[], "ScanOrigin.Z"=w184:sgl)
            n69 = Unbundle By Name(w206) -> ("ScanOrigin.X"=w205:sgl, "ScanOrigin.Y"=w201:sgl)
            n70 = for {
              tunnel: w208 -> [w230] mode=indexing
              tunnel: w184 -> [w229]
              tunnel: "Follow Z offset(mm)" -> [w227]
              tunnel: w193 -> [w223]
              tunnel: w185 -> [w222]
              tunnel: [w221] -> w189 mode=indexing
              tunnel: [w220] -> w187 mode=indexing
              tunnel: [w219] -> w191 mode=indexing
              # "add offset"
              n71 = Unbundle By Name(w230) -> ("x(mm)"=w226:dbl, "y(mm)"=w225:dbl, "z(mm)"=w224:dbl)
              n72 = Add(x=w224, y=w229) -> (x+y=w228:dbl)
              n73 = Add(x=w223, y=w226) -> (x+y=w221:dbl)
              n74 = Add(x=w222, y=w225) -> (x+y=w220:dbl)
              n75 = Add(x=w228, y=w227) -> (x+y=w219:dbl)
            }
            n76 = Add(x=w201, y=w185) -> (x+y=w204:dbl)
            n77 = Add(x=w205, y=w193) -> (x+y=w182:dbl)
            n78 = Subtract(x=w182, y=0.0) -> (x-y=w180:dbl)
            n79 = call "ApplyMaxKernal.vi"("Radius(2mm)"="Probe Radius(2mm)", "Z"=w191, "Y"=w187, "X"=w189) -> ("ZZ"=w190:dbl[])  [unwired: 7 in]
            n80 = call "Go to Position.vi"("X (mm)"=w180, "Speed (2000 mm/min)"=sgl 1500.0 ("Speed (mm/min)"), "Overwright speed? (F)"=TRUE, "Y (mm)"=w204, "Z (mm)"=w184, "error in (no error)"=w179) -> ("error out"=w194:errorcluster)  [unwired: 9 in]
            n81 = flat-sequence {
              tunnel: w194 -> [_]
              frame #0 {
                n82 = One Button Dialog(message="Lower fiber so that it touches the platfom! ", button name ("OK")="Confirm") -> ()  [unwired: 1 out]
              }
            }
            n83 = for {
              tunnel: w190 -> [w210] mode=indexing
              tunnel: w189 -> [w212] mode=indexing
              tunnel: w188 -> [w213]
              tunnel: w187 -> [w211] mode=indexing
              tunnel: [w209] -> w186 mode=indexing
              n84 = Bundle By Name(cluster=w213, "x(mm)"=w212, "y(mm)"=w211, "z(mm)"=w210) -> (w209:cluster{"x(mm)":dbl, "y(mm)":dbl, "z(mm)":dbl})
            }
            n85 = Bundle By Name(cluster=w206, "FollowScan"=w186, "3DProfileToPlot"=w186, "FollowScanZOffset(mm)"="Follow Z offset(mm)", "ProbeRadius(mm)"="Probe Radius(2mm)") -> (w207:T15)
            n86 = property on="Interpolate Scan" class="Bool"(error in=w194, "DisabledEnum"=T6."Enabled" ("Disabled")) -> (error out=w200:errorcluster)  [unwired: 1 in, 1 out]
            n87 = call <vilib>:"Add State(s) to Queue__JKI_lib_State_Machine.vi"("State(s) in Front (\"\")"="LJT4: RestEncoder\nUtility: Plot3D" ("State(s) in Front (\"\")"), "State(s) in (\"\")"=w197) -> ("States Out"=w198:string)  [unwired: 13 in]
          }
          event "Remove Z outlier": Value Change {
            n88 = event-data() -> ()  [unwired: 1 in, 6 out]
            n89 = Unbundle By Name(w240) -> ("Raw3DProfile"=w241:cluster{"x(mm)":dbl, "y(mm)":dbl, "z(mm)":dbl}[])
            n90 = for {
              tunnel: w241 -> [w244] mode=indexing
              tunnel: "Upper Z limite(mm)" -> [w247]
              shift-right: [w245] -> w231
              shift-left: cluster{"x(mm)":dbl, "y(mm)":dbl, "z(mm)":dbl}[] [] -> [w243]
              n91 = Unbundle By Name(w244) -> ("z(mm)"=w248:dbl)
              n92 = Less Or Equal?(x=w248, y=w247) -> (x <= y?=w246:bool)
              n93 = case shown="True" w246 {
                tunnel: [w249 w252] -> w245
                tunnel: w244 -> [_ w251]
                tunnel: w243 -> [w249 w250]
                frame False {
                }
                frame True {
                  n94 = Build Array (concatenate)(w250, w251) -> (w252:cluster{"x(mm)":dbl, "y(mm)":dbl, "z(mm)":dbl}[])
                }
              }
            }
            n95 = property on="Calc follow scan" class="Bool"(error in=w232, "DisabledEnum"=T6."Enabled" ("Disabled")) -> (error out=w233:errorcluster)  [unwired: 1 in, 1 out]
            n96 = Bundle By Name(cluster=w240, "3DProfile"=w231, "3DProfileToPlot"=w231) -> (w239:T15)
            n97 = call <vilib>:"Add State(s) to Queue__JKI_lib_State_Machine.vi"("State(s) in Front (\"\")"="Utility: Plot3D" ("State(s) in Front (\"\")"), "State(s) in (\"\")"=w238) -> ("States Out"=w237:string)  [unwired: 13 in]
          }
          event "Interpolate Scan": Value Change {
            n98 = event-data() -> ()  [unwired: 1 in, 6 out]
            n99 = Unbundle By Name(w266) -> ("FollowScan"=w268:cluster{"x(mm)":dbl, "y(mm)":dbl, "z(mm)":dbl}[])
            n100 = call "InterpRoute.vi"("error in (no error)"=w254, "GridSize(mm)"="FollowScanGridSize(mm)", "FollowScanWOffset"=w268) -> ("error out"=w253:errorcluster, "Zi"=w256:dbl[], "Yi"=w263:dbl[], "Xi"=w264:dbl[])  [unwired: 4 in, 1 out]
            n101 = Index Array(array=w268) -> (element=w267:cluster{"x(mm)":dbl, "y(mm)":dbl, "z(mm)":dbl})  [unwired: 1 in]
            n102 = property on="Follow Scan" class="Bool"(error in=w253, "DisabledEnum"=T6."Enabled" ("Disabled")) -> (error out=w261:errorcluster)  [unwired: 1 in, 1 out]
            n103 = for {
              tunnel: w267 -> [w273]
              tunnel: w264 -> [w272] mode=indexing
              tunnel: w263 -> [w271] mode=indexing
              tunnel: w256 -> [w270] mode=indexing
              tunnel: [w269] -> w257 mode=indexing
              n104 = Bundle By Name(cluster=w273, "x(mm)"=w272, "y(mm)"=w271, "z(mm)"=w270) -> (w269:cluster{"x(mm)":dbl, "y(mm)":dbl, "z(mm)":dbl})
            }
            n105 = Bundle By Name(cluster=w266, "FollowScanWInter"=w257, "3DProfileToPlot"=w257, "FollowGridSize(mm)"="FollowScanGridSize(mm)") -> (w265:T15)
            n106 = call <vilib>:"Add State(s) to Queue__JKI_lib_State_Machine.vi"("State(s) in Front (\"\")"="Utility: Plot3D" ("State(s) in Front (\"\")"), "State(s) in (\"\")"=w259) -> ("States Out"=w258:string)  [unwired: 13 in]
          }
          event "Follow Scan": Value Change {
            w280 = TRUE ("event data")
            w292 = "\r"
            # "set feedrate"
            n107 = event-data() -> ()  [unwired: 1 in, 6 out]
            n108 = call "RemoteEventFGV.vi"() -> ("Remote Event out"=w278:T16)  [unwired: 10 in, 1 out]
            n109 = Unbundle By Name(w278) -> ("remote start event"=w277:refnum<user-event>)
            n110 = Unbundle By Name(w305) -> ("FollowScanWInter"=w287:cluster{"x(mm)":dbl, "y(mm)":dbl, "z(mm)":dbl}[])
            n111 = Generate User Event(priority (normal)=usereventprio."high priority", user event=w277, event data cluster=TRUE ("event data")) -> (error out=w274:errorcluster)  [unwired: 1 in, 1 out]
            n112 = Number To Fractional String(number="Follow Speed (mm/min)", precision (6)=i16 3) -> (F-format string=w301:string)  [unwired: 2 in]
            n113 = Concatenate Strings("F" ("string"), w301, "\r") -> (w300:string)
            n114 = call "Send-Receive Serial Port.vi"("Data to write"=w300, "error in (no error)"=w283) -> ("error out"=w297:errorcluster)  [unwired: 12 in, 1 out]
            n115 = Concatenate Strings("$120=200" ("string"), w292) -> (w291:string)
            n116 = Concatenate Strings("$121=200" ("string"), w292) -> (w290:string)
            n117 = Concatenate Strings("$122=200" ("string"), w292) -> (w289:string)
            n118 = local write "FollowScan"(w280) -> ()
            n119 = Generate User Event(user event=w284, event data cluster=w280, error in=w283) -> (error out=w279:errorcluster)  [unwired: 1 in, 1 out]
            n120 = Build Array(w291, w290, w289) -> (w288:string[])
            n121 = for {
              shift-right: [w307] -> w296
              shift-left: w297 -> [w308]
              tunnel: w288 -> [w306] mode=indexing
              n122 = call "Send-Receive Serial Port.vi"("Data to write"=w306, "error in (no error)"=w308) -> ("error out"=w307:errorcluster)  [unwired: 12 in, 1 out]
            }
            n123 = Generate User Event(user event=w304, event data cluster=w287, error in=w296) -> (error out=w282:errorcluster)  [unwired: 1 in, 1 out]
            n124 = call <vilib>:"Add State(s) to Queue__JKI_lib_State_Machine.vi"("State(s) in (\"\")"=w285) -> ("States Out"=w286:string)  [unwired: 14 in]
            n125 = Merge Errors(w282, w279, w274) -> (w281:errorcluster)
          }
          event "ParseLocationData": Value Change {
            n126 = event-data() -> ()  [unwired: 1 in, 6 out]
            n127 = Unbundle By Name(w317) -> ("ScanOrigin"=w322:cluster{"X":sgl, "Y":sgl, "Z":sgl}, "BG(V)"=w321:dbl, "YPixelSize(mm)"=w319:dbl)
            n128 = Obtain Queue(name (unnamed)="LocationData", element data type=cluster{"Time":dbl, "x":dbl} {"Time"=0.0, "x"=0.0}, error in (no error)=w327) -> (queue out=w328:refnum<queue>, error out=w329:errorcluster)  [unwired: 2 in, 1 out]
            n129 = Flush Queue(queue=w328, error in (no error)=w329) -> (remaining elements=w316:cluster{"Time":dbl, "x":dbl}[], error out=w325:errorcluster)  [unwired: 1 out]
            n130 = for {
              tunnel: w316 -> [w335] mode=indexing
              tunnel: [w333] -> w323 mode=indexing
              n131 = Unbundle By Name(w335) -> ("x"=w332:dbl, "Time"=w331:dbl)
              n132 = Bundle("x"=w332, 0.0, "Time"=w331) -> (w333:cluster{"x":dbl, dbl, "Time":dbl})  [unwired: 1 in]
            }
            n133 = local write "Tab Control"(T2."IntensityGraph" ("Tab Control")) -> ()
            n134 = call "GetPPIXImg.vi"("Background"=w321, "dy"=w319, "Origin"=w322, "3D Profile in"=w323) -> ("Z"=w313:dbl[], "Y"=w314:dbl[], "X"=w315:dbl[])  [unwired: 4 in, 1 out]
            n135 = Bundle("X"=w315, "Y"=w314, "Z"=w313) -> (w312:cluster{"X":dbl[], "Y":dbl[], "Z":dbl[]})  [unwired: 1 in]
            n136 = call-poly <vilib>:"Plot Helper.vi"("z vector"=w313, "y vector"=w314, "x vector"=w315) -> ("3D Plot lvclass Array out"=→"CH1":refnum<class "3D Plot Datatype.lvclass">[])  [unwired: 3 in, 5 out]
            n137 = Bundle By Name(cluster=w317, "RawFollowScanData"=w316, "PPIXProcessedImg"=w312) -> (w318:T15)
            n138 = call <vilib>:"Add State(s) to Queue__JKI_lib_State_Machine.vi"("State(s) in Front (\"\")"="UI: ReadyToSave" ("State(s) in Front (\"\")"), "State(s) in (\"\")"=w311) -> ("States Out"=w310:string)  [unwired: 13 in]
          }
          event "Home": Value Change {
            n139 = event-data() -> ()  [unwired: 1 in, 6 out]
            n140 = call <vilib>:"Add State(s) to Queue__JKI_lib_State_Machine.vi"("State(s) in Front (\"\")"="Stage: Home" ("State(s) in Front (\"\")"), "State(s) in (\"\")"=w338) -> ("States Out"=w339:string)  [unwired: 13 in]
          }
          event "Hault": Value Change {
            n141 = event-data() -> ()  [unwired: 1 in, 6 out]
            n142 = call <vilib>:"Add State(s) to Queue__JKI_lib_State_Machine.vi"("State(s) in Front (\"\")"="Stage: Reset" ("State(s) in Front (\"\")"), "State(s) in (\"\")"=w344) -> ("States Out"=w343:string)  [unwired: 13 in]
          }
          event "X++": Value Change {
            n143 = event-data() -> ()  [unwired: 1 in, 6 out]
            n144 = Unbundle By Name(w356) -> ("StepSize"=w349:dbl)
            n145 = call "Get Status.vi"("error in (no error)"=w346) -> ("Status"=w353:T9, "Current position"=w350:cluster{"X":sgl, "Y":sgl, "Z":sgl}, "error out"=w348:errorcluster)  [unwired: 10 in, 2 out]
            n146 = Equal?(x=Status."Idle" ("Status"), y=w353) -> (x = y?=w351:bool)
            n147 = case shown="True" w351 {
              tunnel: w350 -> [_ w366]
              tunnel: w349 -> [_ w359]
              tunnel: w348 -> [w358 w362]
              tunnel: [w358 w361] -> w347
              frame False {
                n148 = One Button Dialog(message="Stage is not Idle!\nPlease try again when stage is Idle. ") -> ()  [unwired: 1 in, 1 out]
              }
              frame True {
                n149 = Unbundle By Name(w366) -> ("X"=w360:sgl, "Y"=w364:sgl, "Z"=w363:sgl)
                n150 = Add(x=w360, y=w359) -> (x+y=w365:dbl)
                n151 = call "Go to Position.vi"("X (mm)"=w365, "Y (mm)"=w364, "Z (mm)"=w363, "error in (no error)"=w362) -> ("error out"=w361:errorcluster)  [unwired: 11 in]
              }
            }
            n152 = call <vilib>:"Add State(s) to Queue__JKI_lib_State_Machine.vi"("State(s) in (\"\")"=w354) -> ("States Out"=w355:string)  [unwired: 14 in]
          }
          event "Y++": Value Change {
            n153 = event-data() -> ()  [unwired: 1 in, 6 out]
            n154 = Unbundle By Name(w377) -> ("StepSize"=w370:dbl)
            n155 = call "Get Status.vi"("error in (no error)"=w367) -> ("Status"=w374:T9, "Current position"=w371:cluster{"X":sgl, "Y":sgl, "Z":sgl}, "error out"=w369:errorcluster)  [unwired: 10 in, 2 out]
            n156 = Equal?(x=Status."Idle" ("Status"), y=w374) -> (x = y?=w372:bool)
            n157 = case shown="True" w372 {
              tunnel: w371 -> [_ w387]
              tunnel: w370 -> [_ w383]
              tunnel: w369 -> [w379 w385]
              tunnel: [w379 w384] -> w368
              frame False {
                n158 = One Button Dialog(message="Stage is not Idle!\nPlease try again when stage is Idle. ") -> ()  [unwired: 1 in, 1 out]
              }
              frame True {
                n159 = Unbundle By Name(w387) -> ("X"=w380:sgl, "Y"=w382:sgl, "Z"=w386:sgl)
                n160 = Add(x=w382, y=w383) -> (x+y=w381:dbl)
                n161 = call "Go to Position.vi"("X (mm)"=w380, "Y (mm)"=w381, "Z (mm)"=w386, "error in (no error)"=w385) -> ("error out"=w384:errorcluster)  [unwired: 11 in]
              }
            }
            n162 = call <vilib>:"Add State(s) to Queue__JKI_lib_State_Machine.vi"("State(s) in (\"\")"=w375) -> ("States Out"=w376:string)  [unwired: 14 in]
          }
          event "GoToZero": Value Change {
            n163 = event-data() -> ()  [unwired: 1 in, 6 out]
            n164 = call <vilib>:"Add State(s) to Queue__JKI_lib_State_Machine.vi"("State(s) in Front (\"\")"="Stage: GoToZero" ("State(s) in Front (\"\")"), "State(s) in (\"\")"=w389) -> ("States Out"=w390:string)  [unwired: 13 in]
          }
          event "Y--": Value Change {
            n165 = event-data() -> ()  [unwired: 1 in, 6 out]
            n166 = Unbundle By Name(w403) -> ("StepSize"=w396:dbl)
            n167 = call "Get Status.vi"("error in (no error)"=w393) -> ("Status"=w400:T9, "Current position"=w397:cluster{"X":sgl, "Y":sgl, "Z":sgl}, "error out"=w395:errorcluster)  [unwired: 10 in, 2 out]
            n168 = Equal?(x=Status."Idle" ("Status"), y=w400) -> (x = y?=w398:bool)
            n169 = case shown="True" w398 {
              tunnel: w397 -> [_ w413]
              tunnel: w396 -> [_ w409]
              tunnel: w395 -> [w405 w411]
              tunnel: [w405 w410] -> w394
              frame False {
                n170 = One Button Dialog(message="Stage is not Idle!\nPlease try again when stage is Idle. ") -> ()  [unwired: 1 in, 1 out]
              }
              frame True {
                n171 = Unbundle By Name(w413) -> ("X"=w406:sgl, "Y"=w408:sgl, "Z"=w412:sgl)
                n172 = Subtract(x=w408, y=w409) -> (x-y=w407:dbl)
                n173 = call "Go to Position.vi"("X (mm)"=w406, "Y (mm)"=w407, "Z (mm)"=w412, "error in (no error)"=w411) -> ("error out"=w410:errorcluster)  [unwired: 11 in]
              }
            }
            n174 = call <vilib>:"Add State(s) to Queue__JKI_lib_State_Machine.vi"("State(s) in (\"\")"=w401) -> ("States Out"=w402:string)  [unwired: 14 in]
          }
          event "Z--": Value Change {
            n175 = event-data() -> ()  [unwired: 1 in, 6 out]
            n176 = Unbundle By Name(w424) -> ("StepSize"=w417:dbl)
            n177 = call "Get Status.vi"("error in (no error)"=w414) -> ("Status"=w421:T9, "Current position"=w418:cluster{"X":sgl, "Y":sgl, "Z":sgl}, "error out"=w416:errorcluster)  [unwired: 10 in, 2 out]
            n178 = Equal?(x=Status."Idle" ("Status"), y=w421) -> (x = y?=w419:bool)
            n179 = case shown="True" w419 {
              tunnel: w418 -> [_ w434]
              tunnel: w417 -> [_ w431]
              tunnel: w416 -> [w426 w433]
              tunnel: [w426 w432] -> w415
              frame False {
                n180 = One Button Dialog(message="Stage is not Idle!\nPlease try again when stage is Idle. ") -> ()  [unwired: 1 in, 1 out]
              }
              frame True {
                n181 = Unbundle By Name(w434) -> ("X"=w430:sgl, "Y"=w429:sgl, "Z"=w427:sgl)
                n182 = Subtract(x=w427, y=w431) -> (x-y=w428:dbl)
                n183 = call "Go to Position.vi"("X (mm)"=w430, "Y (mm)"=w429, "Z (mm)"=w428, "error in (no error)"=w433) -> ("error out"=w432:errorcluster)  [unwired: 11 in]
              }
            }
            n184 = call <vilib>:"Add State(s) to Queue__JKI_lib_State_Machine.vi"("State(s) in (\"\")"=w422) -> ("States Out"=w423:string)  [unwired: 14 in]
          }
          event "Z++": Value Change {
            n185 = event-data() -> ()  [unwired: 1 in, 6 out]
            n186 = Unbundle By Name(w445) -> ("StepSize"=w438:dbl)
            n187 = call "Get Status.vi"("error in (no error)"=w435) -> ("Status"=w442:T9, "Current position"=w439:cluster{"X":sgl, "Y":sgl, "Z":sgl}, "error out"=w437:errorcluster)  [unwired: 10 in, 2 out]
            n188 = Equal?(x=Status."Idle" ("Status"), y=w442) -> (x = y?=w440:bool)
            n189 = case shown="True" w440 {
              tunnel: w439 -> [_ w455]
              tunnel: w438 -> [_ w452]
              tunnel: w437 -> [w447 w454]
              tunnel: [w447 w453] -> w436
              frame False {
                n190 = One Button Dialog(message="Stage is not Idle!\nPlease try again when stage is Idle. ") -> ()  [unwired: 1 in, 1 out]
              }
              frame True {
                n191 = Unbundle By Name(w455) -> ("X"=w451:sgl, "Y"=w450:sgl, "Z"=w448:sgl)
                n192 = Add(x=w448, y=w452) -> (x+y=w449:dbl)
                n193 = call "Go to Position.vi"("X (mm)"=w451, "Y (mm)"=w450, "Z (mm)"=w449, "error in (no error)"=w454) -> ("error out"=w453:errorcluster)  [unwired: 11 in]
              }
            }
            n194 = call <vilib>:"Add State(s) to Queue__JKI_lib_State_Machine.vi"("State(s) in (\"\")"=w443) -> ("States Out"=w444:string)  [unwired: 14 in]
          }
          event "Set Origin": Value Change {
            # "reset encoder"
            n195 = event-data() -> ()  [unwired: 1 in, 6 out]
            n196 = call "Get Status.vi"("error in (no error)"=w461) -> ("Current position"=w464:cluster{"X":sgl, "Y":sgl, "Z":sgl}, "error out"=w457:errorcluster)  [unwired: 10 in, 3 out]
            "Scan Origin MPos" <- w464
            n197 = call "LabJack_FGV_T4.vi"("Operation(Read)"=enum16{"Write", "Read"}."Read" ("Operation"), "error in (no error)"=w457) -> ("error out"=w460:errorcluster, "Read data"=w459:i32)  [unwired: 8 in]
            n198 = Bundle By Name(cluster=w466, "ScanOrigin"=w464) -> (w465:T15)
            n199 = call "LJM_eReadName.vi"("Handle In"=w459, "Name"="DIO4_EF_READ_A_AND_RESET", "error in"=w460) -> ("error out"=w456:errorcluster)  [unwired: 10 in, 2 out]
          }
          event "3DProfileScan": Value Change {
            n200 = event-data() -> ()  [unwired: 1 in, 6 out]
            n201 = One Button Dialog(message="Please raise fiber!", button name ("OK")="Confirm!") -> (true=w467:bool)
            n202 = case shown="True" w467 {
              tunnel: w476 -> [_ w504]
              tunnel: w475 -> [w481 w503]
              tunnel: [w480 w496] -> w474
              tunnel: w473 -> [w480 w495]
              tunnel: ["" ("State(s) in Front (\"\")") "AccuRange: Start" ("State(s) in Front (\"\")")] -> w472
              tunnel: w471 -> [_ w488]
              tunnel: [w481 w485] -> w470
              frame False {
              }
              frame True {
                # "set feedrate"
                # "Flush queue"
                n203 = Unbundle By Name(w495) -> ("ScanOrigin"=w505:cluster{"X":sgl, "Y":sgl, "Z":sgl})
                n204 = Flush Queue(queue=w504, error in (no error)=w503) -> (error out=w502:errorcluster)  [unwired: 2 out]
                n205 = call "RoutePlaner.vi"("Origin In"=w505, "Pixel Size(mm)"="Y Pixel Size(mm)", "Y distance(mm)"="Y distance(mm)", "X distance (mm)"="X distance (mm)") -> ("TotalDistance (mm)"=w493:dbl, "PtArray"=w487:cluster{"x":dbl, "y":dbl, "z":dbl}[])  [unwired: 5 in, 1 out]
                n206 = Number To Fractional String(number="Pre Scan Speed\n(mm/min)", precision (6)=i16 3) -> (F-format string=w499:string)  [unwired: 2 in]
                n207 = Divide(x=w493, y="Pre Scan Speed\n(mm/min)") -> (x/y=w491:dbl)
                n208 = Multiply(x=w491, y=60.0) -> (x*y=w484:dbl)
                n209 = Concatenate Strings("F" ("string"), w499, "\r") -> (w498:string)
                n210 = Add(x=w484, y=10.0) -> (x+y=→"Estimated surface\n scan time (s)":dbl)
                n211 = call "Send-Receive Serial Port.vi"("Data to write"=w498, "error in (no error)"=w502) -> ("error out"=w486:errorcluster)  [unwired: 12 in, 1 out]
                n212 = Bundle By Name(cluster=w495, "YPixelSize(mm)"="Y Pixel Size(mm)") -> (w496:T15)
                n213 = Generate User Event(user event=w488, event data cluster=w487, error in=w486) -> (error out=w485:errorcluster)  [unwired: 1 in, 1 out]
              }
            }
            n214 = call <vilib>:"Add State(s) to Queue__JKI_lib_State_Machine.vi"("State(s) in Front (\"\")"=w472, "State(s) in (\"\")"=w478) -> ("States Out"=w477:string)  [unwired: 13 in]
          }
          event "AbortScan": Value Change {
            n215 = event-data() -> ()  [unwired: 1 in, 6 out]
            "AbortFlag" <- "AbortScan"
          }
          event "X--": Value Change {
            n216 = event-data() -> ()  [unwired: 1 in, 6 out]
            n217 = Unbundle By Name(w522) -> ("StepSize"=w515:dbl)
            n218 = call "Get Status.vi"("error in (no error)"=w512) -> ("Status"=w519:T9, "Current position"=w516:cluster{"X":sgl, "Y":sgl, "Z":sgl}, "error out"=w514:errorcluster)  [unwired: 10 in, 2 out]
            n219 = Equal?(x=Status."Idle" ("Status"), y=w519) -> (x = y?=w517:bool)
            n220 = case shown="True" w517 {
              tunnel: w516 -> [_ w532]
              tunnel: w515 -> [_ w526]
              tunnel: w514 -> [w524 w528]
              tunnel: [w524 w527] -> w513
              frame False {
                n221 = One Button Dialog(message="Stage is not Idle!\nPlease try again when stage is Idle. ") -> ()  [unwired: 1 in, 1 out]
              }
              frame True {
                n222 = Unbundle By Name(w532) -> ("X"=w525:sgl, "Y"=w530:sgl, "Z"=w529:sgl)
                n223 = Subtract(x=w525, y=w526) -> (x-y=w531:dbl)
                n224 = call "Go to Position.vi"("X (mm)"=w531, "Y (mm)"=w530, "Z (mm)"=w529, "error in (no error)"=w528) -> ("error out"=w527:errorcluster)  [unwired: 11 in]
              }
            }
            n225 = call <vilib>:"Add State(s) to Queue__JKI_lib_State_Machine.vi"("State(s) in (\"\")"=w520) -> ("States Out"=w521:string)  [unwired: 14 in]
          }
          event "Jog Step Size(mm)": Value Change {
            n226 = event-data() -> ("NewVal"=w534:dbl)  [unwired: 1 in, 5 out]
            n227 = Bundle By Name(cluster=w537, "StepSize"=w534) -> (w536:T15)
          }
          event "Quit": Value Change {
            # "Exit Button Value Change (pressed) Event\n(this executes Macro: Exit to terminate the VI)"
            n228 = event-data() -> ()  [unwired: 1 in, 1 out]
            n229 = call <vilib>:"Add State(s) to Queue__JKI_lib_State_Machine.vi"("State(s) in Front (\"\")"="Macro: Exit", "State(s) in (\"\")"=w542) -> ("States Out"=w541:string)  [unwired: 13 in]
          }
          event "Start": Value Change {
            n230 = event-data() -> ()  [unwired: 1 in, 6 out]
            n231 = call <vilib>:"Add State(s) to Queue__JKI_lib_State_Machine.vi"("State(s) in Front (\"\")"="AccuRange: Start" ("State(s) in Front (\"\")"), "State(s) in (\"\")"=w546) -> ("States Out"=w545:string)  [unwired: 13 in]
          }
          event "Stop": Value Change {
            n232 = event-data() -> ()  [unwired: 1 in, 6 out]
            n233 = call <vilib>:"Add State(s) to Queue__JKI_lib_State_Machine.vi"("State(s) in Front (\"\")"="AccuRange: Stop" ("State(s) in Front (\"\")"), "State(s) in (\"\")"=w551) -> ("States Out"=w550:string)  [unwired: 13 in]
          }
          event Panel Close? {
            # "Discard the event because we'll close the front panel ourselves in Macro: Exit"
            # "Close Panel button (pressed) Event\n(this executes Macro: Exit to terminate the VI)"
            n234 = event-data() -> ()  [unwired: 1 in, 1 out]
            n235 = call <vilib>:"Add State(s) to Queue__JKI_lib_State_Machine.vi"("State(s) in Front (\"\")"="Macro: Exit", "State(s) in (\"\")"=w558) -> ("States Out"=w557:string)  [unwired: 13 in]
            n236 = event-data("Discard?"=TRUE) -> ()  [unwired: 1 in, 1 out]
          }
        }
      }
      frame "---------- Macro ----------" {
        # "Do not put any code in this frame.\n(It is a separator no-op. You can make a copy of this frame to create a new Macro frame)"
        n237 = call <vilib>:"Add State(s) to Queue__JKI_lib_State_Machine.vi"("State(s) in (\"\")"=w563) -> ("States Out"=w562:string)  [unwired: 14 in]
      }
      frame "Macro: Initialize" {
        # "Initialization Macro\n(This is called once, when the VI starts)"
        n238 = call <vilib>:"Add State(s) to Queue__JKI_lib_State_Machine.vi"("State(s) in Front (\"\")"="Data: Initialize\nInitialize Core Data\nUI: Initialize\nUI: Front Panel State >> Open\nData: UpdateStepSize\nUI: StartUp\nUI: Cursor Set >> Busy\nStage: Initialize\nUI: Update\nAccuRange: Initialize\nUI: Update\nLJT4: Initialize\nUI: Update\n/*USBCam: Initialize\nLJT4: Config\nStage: Reset\nStage: Config\nAccuRange: Config\nAccuRange: Start\nData: CreatDataFolder\nUI: Cursor Set >> Idle\nStage: Home\nStage: GoToZero\nUI: Update", "State(s) in (\"\")"=w564) -> ("States Out"=w569:string)  [unwired: 13 in]
      }
      frame "Macro: SaveData" {
        # "Save 3D profile and scan data\n()"
        n239 = call <vilib>:"Add State(s) to Queue__JKI_lib_State_Machine.vi"("State(s) in Front (\"\")"="Data: OpenTDMS\nData: SaveExpDetail\nData: SaveRaw3DProfile\nData: SaveProcessed3DProfile\nData: SaveFollowScan\nData: SaveInterpedFollowScan\nData: SaveRawFollowScanData\nData: SaveProcessedPPIXImg\nData: CloseTDMS\nDialog: DataSaved" ("State(s) in Front (\"\")"), "State(s) in (\"\")"=w575) -> ("States Out"=w574:string)  [unwired: 13 in]
      }
      frame "Macro: Exit" {
        # "Exit Macro\n(This is called once, when the VI exits)"
        n240 = Unbundle By Name(w584) -> ("Core.Close Panel on Exit?"=w583:bool)
        n241 = Select(t="UI: Front Panel State >> Close", s=w583, f="") -> (s? t:f=w580:string)
        n242 = call <vilib>:"Add State(s) to Queue__JKI_lib_State_Machine.vi"("State(s) in Front (\"\")"="AccuRange: Stop\nStage: Close\nAccuRange: Close\nLJT4: Close\n/*USBCam: Close\nUI: Update\nUtility: DestroyQueue" ("State(s) in Front (\"\")"), "State(s) in (\"\")"=w580, "State(s) at Back (\"\")"="Data: Cleanup\nExit") -> ("States Out"=w578:string)  [unwired: 12 in]
        n243 = call <vilib>:"Add State(s) to Queue__JKI_lib_State_Machine.vi"("State(s) in Front (\"\")"=w578, "State(s) in (\"\")"=w587) -> ("States Out"=w586:string)  [unwired: 13 in]
      }
      frame "---------- Core ----------" {
        # "Do not put any code in this frame.\n(it is a separator no-op)"
        n244 = call <vilib>:"Add State(s) to Queue__JKI_lib_State_Machine.vi"("State(s) in (\"\")"=w592) -> ("States Out"=w591:string)  [unwired: 14 in]
      }
      frame Default {
        w603 = 42 items=["No error", "Argument error", "Memory is full", "Out of zone", "End of file", "File already open", "Generic file I/O error", "File not found", "File permission error", "Disk is full", "Duplicate path", "Too many files open", "System feature not enabled", "Resource file not found", "Cannot add resource", "Resource not found", "Image not found", "Image memory error", "Pen does not exist", "Config type invalid", "Config token not found", "Config parse error", "Config memory error", "Bad external code format", "Bad external code offset", "External code not present", "Null window", "Destroy window error", "Null menu", "Print aborted", "Bad print record", "Print driver error", "Windows error during printing", "Memory error during printing", "Print dialog error", "Generic print error", "Invalid device refnum", "Device not found", "Device parameter error", "Device unit error", "Cannot open device", "Device call aborted", "Generic error", "Cancelled by user", "Object ID too low", "Object ID too high", "Object not in heap", "Unknown heap", "Unknown object (invalid DefProc)", "Unknown object (DefProc not in table)", "Message out of range", "Invalid (null) method", "Unknown message", "Manager call not supported", "Bad address", "Network operation in progress", "Network operation timed out", "Connection is busy", "Network attribute not supported", "Network error", "Address in use", "System out of memory", "Connection aborted", "Connection refused", "Not connected", "Already connected", "Connection closed", "Initialization error (interapplication manager)", "Bad occurrence", "Wait on unbound occurrence handler", "Occurrence queue overflow", "Datalog type conflict", "Unused", "Unrecognized type (interapplication manager)", "Memory corrupt", "Failed to make temporary DLL", "Old CIN version", "Drag socket not found", "Failed to load drop-object", "Failed to register OLE object", "Failed to release OLE object", "Format specifier type mismatch", "Unknown format specifier", "Too few format specifiers", "Too many format specifiers", "Scan failed", "Newer CIN version", "Error converting to variant", "Runtime menu error", "Password tampered", "Variant attribute not found", "Incompatible variant data type", "Event data is not available", "Event Store is not present", "Occurrence is not found", "Event Queue is not created", "Event info is not available", "Refnum passed is NULL", "Error retrieving Class GUID", "Error retrieving CoClass GUID", "Error retrieving TypeLib GUID.", "Bad built application magic bytes.", "Specific driver is different from the specific driver associated with the Logical Name.", "There is no session opened to the class driver.", "Max Error", "MAX - Error with config objects", "MAX - Error loading configuration", "MAX - Group not supported"]
        # "Current State"
        # "Do not delete, rename, or modify this frame.\n(this is used to capture unhandled states and typos)"
        # "Handle mistyped state name (developer tool)"
        n245 = Format Into String(format string="Software Exception: Unhandled State \"%s\"." ("message"), error in=w599, w594) -> (resulting string=w602:string, error out=w601:errorcluster)  [unwired: 1 in]
        n246 = call <vilib>:"Error Cluster From Error Code.vi"("show call chain? (False)"=TRUE, "error in (no error)"=w601, "error message (\"\")"=w602, "error code (0)"=w603) -> ("error out"=w600:errorcluster)  [unwired: 5 in]
        n247 = call <vilib>:"Add State(s) to Queue__JKI_lib_State_Machine.vi"("State(s) in (\"\")"=w598) -> ("States Out"=w597:string)  [unwired: 14 in]
      }
      frame "Initialize Core Data" {
        # "Do not delete, rename, or modify this frame.\n(this is used to determine panel behavior on exit)"
        # "originally closed?"
        # "exe?"
        # "If panel starts closed or is an EXE, then close it when we exit"
        n248 = property class="VI"() -> ("FP.State"=w608:T10)  [unwired: 2 in, 2 out]
        n249 = property class="App"() -> ("App.Kind"=w614:T11)  [unwired: 2 in, 2 out]
        n250 = control-ref of="Current VI Reference"() -> (w609:refnum<vi>)
        n251 = Equal?(x=w608, y=T10."Closed" ("Front Panel Window:State")) -> (x = y?=w606:bool)
        n252 = Equal?(x=w614, y=T11."Run Time System" ("Application:Kind")) -> (x = y?=w612:bool)
        n253 = Or(x=w606, y=w612) -> (x .or. y?=w610:bool)
        n254 = Bundle By Name(cluster=w611, "Core.Current VI Reference"=w609, "Core.Close Panel on Exit?"=w610) -> (w616:T15)
        n255 = call <vilib>:"Add State(s) to Queue__JKI_lib_State_Machine.vi"("State(s) in (\"\")"=w618) -> ("States Out"=w617:string)  [unwired: 14 in]
      }
      frame "Error Handler" {
        # "Unhandled Error -- Display it"
        # "Handle any errors here.\nYou can also output any states to clean-up after errors occur"
        # "Clear error"
        n256 = call <vilib>:"General Error Handler.vi"("error in (no error)"=w621) -> ()  [unwired: 10 in, 5 out]
        n257 = call <vilib>:"Add State(s) to Queue__JKI_lib_State_Machine.vi"("State(s) in Front (\"\")"="/* Post Error States\nMacro: Exit", "State(s) in (\"\")"=w625) -> ("States Out"=w624:string)  [unwired: 13 in]
      }
      frame "Exit" {
        # "Do not put any code in this frame.\n(No errors that occur here will be handled.)"
        n258 = Generate User Event(user event=w629, event data cluster=TRUE ("event data"), error in=w627) -> (error out=w628:errorcluster)  [unwired: 1 in, 1 out]
        n259 = call <vilib>:"Add State(s) to Queue__JKI_lib_State_Machine.vi"("State(s) in (\"\")"=w634) -> ("States Out"=w633:string)  [unwired: 14 in]
      }
      frame "---------- Data ----------" {
        # "Do not put any code in this frame.\n(It is a separator no-op. You can make a copy of this frame to create a new Data frame)"
        n260 = call <vilib>:"Add State(s) to Queue__JKI_lib_State_Machine.vi"("State(s) in (\"\")"=w639) -> ("States Out"=w638:string)  [unwired: 14 in]
      }
      frame "Data: Initialize" {
        w640 = 0.0  # FollowGridSize(mm)
        w641 = 0.0  # ProbeRadius(mm)
        w642 = cluster{"x":dbl[], "y":dbl[], "Time(ms)":dbl[]} {"x"=[], "y"=[], "Time(ms)"=[]}  # PPIXProcessedImg
        w643 = cluster{"Time(ms)":dbl, "x":dbl}[] []  # RawFollowScanData
        w644 = 0.0  # FollowScanZOffset(mm)
        w645 = cluster{"x":dbl, "y":dbl} {"x"=-21.5, "y"=-70.0}  # FiberOffset
        w646 = refnum<k34> refnum  # tdms file
        w647 = cluster{"x(mm)":dbl, "y(mm)":dbl, "z(mm)":dbl}[] []  # Raw3DProfileNoY
        w648 = path ""  # SaveFilePath
        w649 = cluster{"x(mm)":dbl, "y(mm)":dbl, "z(mm)":dbl}[] []  # FollowScan
        w650 = cluster{"x(mm)":dbl, "y(mm)":dbl, "z(mm)":dbl}[] []  # 3DProfileToPlot
        w653 = cluster{"X":sgl, "Y":sgl, "Z":sgl} {"X"=0.0, "Y"=0.0, "Z"=0.0}  # HomeMposOrigin
        w654 = FALSE  # StageHomed?
        w655 = 0.0  # BG(V)
        w656 = cluster{"x(mm)":dbl, "y(mm)":dbl, "z(mm)":dbl}[] []  # FollowScanWInter
        w657 = 0.0  # YPixelSize(mm)
        w658 = cluster{"x(mm)":dbl, "y(mm)":dbl, "z(mm)":dbl}[] []  # Raw3DProfile
        w659 = cluster{"x(mm)":dbl, "y(mm)":dbl, "z(mm)":dbl}[] []  # 3DProfile
        w660 = T4 refnum  # USBCam
        w661 = T5 refnum  # IMAQ
        w662 = 0  # Tic
        w663 = cluster{"X":sgl, "Y":sgl, "Z":sgl} {"X"=0.0, "Y"=0.0, "Z"=0.0}  # ScanOrigin
        w664 = 5.0  # StepSize
        w665 = refnum<visa-resource-name> "COM5"  # RangeCOM
        w666 = refnum<visa-resource-name> "COM3"  # StageCOM
        w652 = T1 {"Stage"=FALSE, "T4"=FALSE, "RangerFinder"=FALSE, "USB Cam"=FALSE}  # Sys Status
        w667 = T17 {"Current VI Reference"=refnum, "Close Panel on Exit?"=FALSE}  # Core
        # "Initialize the shift-register data, here.\n(data names are defined by what you wire into the bundle function)"
        n261 = Bundle("Core"=w667, "Sys Status"=w652, "StageCOM"=w666, "RangeCOM"=w665, "StepSize"=w664, "ScanOrigin"=w663, "HomeMposOrigin"=w653, "Tic"=w662, "IMAQ"=w661, "USBCam"=w660, "3DProfile"=w659, "Raw3DProfile"=w658, "FollowScanZOffset(mm)"=w644, "YPixelSize(mm)"=w657, "FollowScanWInter"=w656, "BG(V)"=w655, "StageHomed?"=w654, "3DProfileToPlot"=w650, "FollowScan"=w649, "SaveFilePath"=w648, "Raw3DProfileNoY"=w647, "tdms file"=w646, "FiberOffset"=w645, "RawFollowScanData"=w643, "PPIXProcessedImg"=w642, "ProbeRadius(mm)"=w641, "FollowGridSize(mm)"=w640) -> (w669:T15)  [unwired: 1 in]
        n262 = call <vilib>:"Add State(s) to Queue__JKI_lib_State_Machine.vi"("State(s) in (\"\")"=w671) -> ("States Out"=w670:string)  [unwired: 14 in]
      }
      frame "Data: UpdateStepSize" {
        # "Template Separator\n(You can make a copy of, or modify, this frame)"
        n263 = Bundle By Name(cluster=w674, "StepSize"="Jog Step Size(mm)") -> (w675:T15)
        n264 = call <vilib>:"Add State(s) to Queue__JKI_lib_State_Machine.vi"("State(s) in (\"\")"=w678) -> ("States Out"=w677:string)  [unwired: 14 in]
      }
      frame "Data: Cleanup" {
        # "Cleanup any data and references, here.\n(this is called automatically, by the Macro: Exit)"
        n265 = Unbundle By Name(w680) -> ("Core.Current VI Reference"=w683:refnum<vi>)
        n266 = Close Reference(reference=w683, error in (no error)=w682) -> (error out=w681:errorcluster)
        n267 = call <vilib>:"Add State(s) to Queue__JKI_lib_State_Machine.vi"("State(s) in (\"\")"=w685) -> ("States Out"=w684:string)  [unwired: 14 in]
      }
      frame "Data: OpenTDMS" {
        # "Open tdms file and save ref num\n(It is a separator no-op. You can make a copy of this frame to create a new Data frame)"
        n268 = call "RunIDFGV.vi"("action (write)"=enum16{"write", "read"}."read") -> ("RunID out"=w695:u16)  [unwired: 9 in, 1 out]
        n269 = Increment(x=w695) -> (x+1=w689:u16)
        n270 = Unbundle By Name(w702) -> ("SaveFilePath"=w693:path)
        n271 = Format Value(format string="%03d", value (0)=w689) -> (output string=w687:string)  [unwired: 1 in]
        n272 = Get Date/Time In Seconds() -> (seconds since 1Jan1904=w699:timestamp)
        n273 = Format Date/Time String(time format string (%c)="%Y%m%d %H_%M", seconds (now)=w699) -> (date/time string=w694:string)  [unwired: 1 in]
        n274 = call <vilib>:"Space Constant.vi"() -> ("String"=w686:string)
        n275 = Concatenate Strings("Run" ("string"), w687, w686, w694, ".tdms" ("string")) -> (w692:string)
        n276 = Build Path(base path=w693, name or relative path=w692) -> (appended path=w690:path)
        n277 = TDMS Open(8:w703, 10:T12."create" ("operation (0:open)"), 11:w690) -> (0:w704:errorcluster, 3:w700:refnum<k34>)  [unwired: 4 in]
        n278 = Bundle By Name(cluster=w702, "tdms file"=w700) -> (w701:T15)
        n279 = call <vilib>:"Add State(s) to Queue__JKI_lib_State_Machine.vi"("State(s) in (\"\")"=w708) -> ("States Out"=w707:string)  [unwired: 14 in]
      }
      frame "Data: SaveExpDetail" {
        # "Save 3D profile to tdms file\n(save y pixel size, raw 3D profile and processed 3D profile to file)"
        n280 = Unbundle By Name(w718) -> ("tdms file"=w717:refnum<k34>)
        n281 = TDMS Set Properties(5:"FLIm 3D Scan", 7:"System", 8:w716, 11:w717) -> (0:w712:errorcluster, 3:w713:refnum<k34>)  [unwired: 2 in, 2 out]
        n282 = Get Date/Time In Seconds() -> (seconds since 1Jan1904=w710:timestamp)
        n283 = TDMS Set Properties(5:w710, 7:"datetime", 8:w712, 11:w713) -> (0:w711:errorcluster)  [unwired: 2 in, 3 out]
        n284 = call <vilib>:"Add State(s) to Queue__JKI_lib_State_Machine.vi"("State(s) in (\"\")"=w721) -> ("States Out"=w720:string)  [unwired: 14 in]
      }
      frame "Data: SaveRaw3DProfile" {
        # "Save 3D profile to tdms file\n(save y pixel size, raw 3D profile and processed 3D profile to file)"
        n285 = Unbundle By Name(w746) -> ("tdms file"=w728:refnum<k34>, "Raw3DProfileNoY"=w743:cluster{"x(mm)":dbl, "y(mm)":dbl, "z(mm)":dbl}[], "YPixelSize(mm)"=w736:dbl)
        n286 = for {
          tunnel: w743 -> [w752] mode=indexing
          tunnel: [w751] -> w742 mode=indexing
          tunnel: [w750] -> w741 mode=indexing
          n287 = Unbundle By Name(w752) -> ("x(mm)"=w751:dbl, "z(mm)"=w750:dbl)
        }
        n288 = Build Array(w742, w741) -> (w740:dbl[][])
        n289 = TDMS Write(0:w728, 5:"Raw3DProfile" ("group name in (Untitled)"), 7:string[] ["x", "z"] ("channel name(s) in (Untitled)"), 9:w740, 11:w729) -> (4:w739:refnum<k34>, 6:w738:string, 15:w735:errorcluster)  [unwired: 1 in, 1 out]
        n290 = TDMS Set Properties(5:w736, 7:"Y pixel size", 8:w735, 10:w738, 11:w739) -> (0:w733:errorcluster, 2:w732:string, 3:w734:refnum<k34>)  [unwired: 1 in, 1 out]
        n291 = local read "Pre Scan Speed\n(mm/min)"() -> (w723:sgl)
        n292 = TDMS Set Properties(5:"mm", 7:"unit", 8:w733, 10:w732, 11:w734) -> (0:w726:errorcluster, 2:w725:string, 3:w727:refnum<k34>)  [unwired: 1 in, 1 out]
        n293 = TDMS Set Properties(5:w723, 7:"ScanSpeed(mm/min)", 8:w726, 10:w725, 11:w727) -> (0:w722:errorcluster)  [unwired: 1 in, 3 out]
        n294 = call <vilib>:"Add State(s) to Queue__JKI_lib_State_Machine.vi"("State(s) in (\"\")"=w749) -> ("States Out"=w748:string)  [unwired: 14 in]
      }
      frame "Data: SaveProcessed3DProfile" {
        # "Save 3D profile to tdms file\n(save y pixel size, raw 3D profile and processed 3D profile to file)"
        n295 = Unbundle By Name(w768) -> ("tdms file"=w754:refnum<k34>, "3DProfile"=w765:cluster{"x(mm)":dbl, "y(mm)":dbl, "z(mm)":dbl}[])
        n296 = for {
          tunnel: w765 -> [w775] mode=indexing
          tunnel: [w774] -> w764 mode=indexing
          tunnel: [w773] -> w763 mode=indexing
          tunnel: [w772] -> w753 mode=indexing
          n297 = Unbundle By Name(w775) -> ("x(mm)"=w774:dbl, "y(mm)"=w773:dbl, "z(mm)"=w772:dbl)
        }
        n298 = Build Array(w764, w763, w753) -> (w762:dbl[][])
        n299 = TDMS Write(0:w754, 5:"Processed3DProfile" ("group name in (Untitled)"), 7:string[] ["x", "y", "z"] ("channel name(s) in (Untitled)"), 9:w762, 11:w755) -> (4:w761:refnum<k34>, 6:w760:string, 15:w759:errorcluster)  [unwired: 1 in, 1 out]
        n300 = TDMS Set Properties(5:"mm", 7:"unit", 8:w759, 10:w760, 11:w761) -> (0:w756:errorcluster)  [unwired: 1 in, 3 out]
        n301 = call <vilib>:"Add State(s) to Queue__JKI_lib_State_Machine.vi"("State(s) in (\"\")"=w771) -> ("States Out"=w770:string)  [unwired: 14 in]
      }
      frame "Data: SaveFollowScan" {
        # "Save 3D profile to tdms file\n(save y pixel size, raw 3D profile and processed 3D profile to file)"
        n302 = Unbundle By Name(w809) -> ("tdms file"=w796:refnum<k34>, "FollowScan"=w806:cluster{"x(mm)":dbl, "y(mm)":dbl, "z(mm)":dbl}[], "FiberOffset"=w790:cluster{"x":dbl, "y":dbl}, "FollowScanZOffset(mm)"=w782:dbl, "ProbeRadius(mm)"=w777:dbl)
        n303 = for {
          tunnel: w806 -> [w816] mode=indexing
          tunnel: [w815] -> w805 mode=indexing
          tunnel: [w814] -> w804 mode=indexing
          tunnel: [w813] -> w795 mode=indexing
          n304 = Unbundle By Name(w816) -> ("x(mm)"=w815:dbl, "y(mm)"=w814:dbl, "z(mm)"=w813:dbl)
        }
        n305 = Build Array(w805, w804, w795) -> (w803:dbl[][])
        n306 = TDMS Write(0:w796, 5:"FollowScan3D" ("group name in (Untitled)"), 7:string[] ["x", "y", "z"] ("channel name(s) in (Untitled)"), 9:w803, 11:w797) -> (4:w802:refnum<k34>, 6:w801:string, 15:w800:errorcluster)  [unwired: 1 in, 1 out]
        n307 = Unbundle By Name(w790) -> ("x"=w789:dbl, "y"=w788:dbl)
        n308 = TDMS Set Properties(5:"mm", 7:"unit", 8:w800, 10:w801, 11:w802) -> (0:w792:errorcluster, 2:w793:string, 3:w794:refnum<k34>)  [unwired: 1 in, 1 out]
        n309 = Build Array(w789, w788) -> (w787:dbl[])
        n310 = TDMS Set Properties(5:w787, 7:string[] ["FiberOffSetX", "FiberOffSetY"] ("property names"), 8:w792, 10:w793, 11:w794) -> (0:w785:errorcluster, 2:w784:string, 3:w786:refnum<k34>)  [unwired: 1 in, 1 out]
        n311 = TDMS Set Properties(5:w782, 7:"FollowOffsetZ", 8:w785, 10:w784, 11:w786) -> (0:w780:errorcluster, 2:w779:string, 3:w781:refnum<k34>)  [unwired: 1 in, 1 out]
        n312 = TDMS Set Properties(5:w777, 7:"ProbeRadius", 8:w780, 10:w779, 11:w781) -> (0:w776:errorcluster)  [unwired: 1 in, 3 out]
        n313 = call <vilib>:"Add State(s) to Queue__JKI_lib_State_Machine.vi"("State(s) in (\"\")"=w812) -> ("States Out"=w811:string)  [unwired: 14 in]
      }
      frame "Data: SaveInterpedFollowScan" {
        # "Save 3D profile to tdms file\n(save y pixel size, raw 3D profile and processed 3D profile to file)"
        n314 = Unbundle By Name(w837) -> ("tdms file"=w824:refnum<k34>, "FollowScanWInter"=w834:cluster{"x(mm)":dbl, "y(mm)":dbl, "z(mm)":dbl}[], "FollowGridSize(mm)"=w818:dbl)
        n315 = for {
          tunnel: w834 -> [w844] mode=indexing
          tunnel: [w843] -> w833 mode=indexing
          tunnel: [w842] -> w832 mode=indexing
          tunnel: [w841] -> w823 mode=indexing
          n316 = Unbundle By Name(w844) -> ("x(mm)"=w843:dbl, "y(mm)"=w842:dbl, "z(mm)"=w841:dbl)
        }
        n317 = Build Array(w833, w832, w823) -> (w831:dbl[][])
        n318 = TDMS Write(0:w824, 5:"InterpedFollowScan3D" ("group name in (Untitled)"), 7:string[] ["x", "y", "z"] ("channel name(s) in (Untitled)"), 9:w831, 11:w825) -> (4:w830:refnum<k34>, 6:w829:string, 15:w828:errorcluster)  [unwired: 1 in, 1 out]
        n319 = TDMS Set Properties(5:"mm", 7:"unit", 8:w828, 10:w829, 11:w830) -> (0:w820:errorcluster, 2:w821:string, 3:w822:refnum<k34>)  [unwired: 1 in, 1 out]
        n320 = TDMS Set Properties(5:w818, 7:"GridSize(mm)", 8:w820, 10:w821, 11:w822) -> (0:w817:errorcluster)  [unwired: 1 in, 3 out]
        n321 = call <vilib>:"Add State(s) to Queue__JKI_lib_State_Machine.vi"("State(s) in (\"\")"=w840) -> ("States Out"=w839:string)  [unwired: 14 in]
      }
      frame "Data: SaveRawFollowScanData" {
        # "Save 3D profile to tdms file\n(save y pixel size, raw 3D profile and processed 3D profile to file)"
        n322 = Unbundle By Name(w869) -> ("tdms file"=w861:refnum<k34>, "RawFollowScanData"=w866:cluster{"Time(ms)":dbl, "x":dbl}[], "YPixelSize(mm)"=w857:dbl)
        n323 = for {
          tunnel: w866 -> [w875] mode=indexing
          tunnel: [w874] -> w865 mode=indexing
          tunnel: [w873] -> w864 mode=indexing
          n324 = Unbundle By Name(w875) -> ("x"=w874:dbl, "Time(ms)"=w873:dbl)
        }
        n325 = Build Array(w865, w864) -> (w863:dbl[][])
        n326 = TDMS Write(0:w861, 5:"RawFollowScanData" ("group name in (Untitled)"), 7:string[] ["x", "Time(ms)", ""] ("channel name(s) in (Untitled)"), 9:w863, 11:w862) -> (4:w860:refnum<k34>, 6:w859:string, 15:w858:errorcluster)  [unwired: 1 in, 1 out]
        n327 = local read "Follow Speed (mm/min)"() -> (w851:sgl)
        n328 = TDMS Set Properties(5:w857, 7:"Y pixel size", 8:w858, 10:w859, 11:w860) -> (0:w854:errorcluster, 2:w853:string, 3:w855:refnum<k34>)  [unwired: 1 in, 1 out]
        n329 = local read "LocationPollingStart"() -> (w845:u32)
        n330 = TDMS Set Properties(5:w851, 7:"ScanSpeed(mm/min)", 8:w854, 10:w853, 11:w855) -> (0:w849:errorcluster, 2:w846:string, 3:w850:refnum<k34>)  [unwired: 1 in, 1 out]
        n331 = TDMS Set Properties(5:w845, 7:"FollowScanStartTime", 8:w849, 10:w846, 11:w850) -> (0:w848:errorcluster)  [unwired: 1 in, 3 out]
        n332 = call <vilib>:"Add State(s) to Queue__JKI_lib_State_Machine.vi"("State(s) in (\"\")"=w872) -> ("States Out"=w871:string)  [unwired: 14 in]
      }
      frame "Data: SaveProcessedPPIXImg" {
        # "Save 3D profile to tdms file\n(save y pixel size, raw 3D profile and processed 3D profile to file)"
        n333 = Unbundle By Name(w886) -> ("tdms file"=w881:refnum<k34>, "PPIXProcessedImg"=w879:cluster{"x":dbl[], "y":dbl[], "Time(ms)":dbl[]})
        n334 = Unbundle By Name(w879) -> ("x"=w876:dbl[], "y"=w878:dbl[], "Time(ms)"=w877:dbl[])
        n335 = Build Array(w876, w878, w877) -> (w883:dbl[][])
        n336 = TDMS Write(0:w881, 5:"ProcessedFollowScanData" ("group name in (Untitled)"), 7:string[] ["x", "y", "Time(ms)"] ("channel name(s) in (Untitled)"), 9:w883, 11:w882) -> (15:w880:errorcluster)  [unwired: 1 in, 3 out]
        n337 = call <vilib>:"Add State(s) to Queue__JKI_lib_State_Machine.vi"("State(s) in (\"\")"=w889) -> ("States Out"=w888:string)  [unwired: 14 in]
      }
      frame "Data: CloseTDMS" {
        # "Close tfms file.\n(It is a separator no-op. You can make a copy of this frame to create a new Data frame)"
        n338 = Unbundle By Name(w893) -> ("tdms file"=w892:refnum<k34>)
        n339 = TDMS Close(8:w890, 11:w892) -> (0:w891:errorcluster)  [unwired: 1 out]
        n340 = call <vilib>:"Add State(s) to Queue__JKI_lib_State_Machine.vi"("State(s) in (\"\")"=w896) -> ("States Out"=w895:string)  [unwired: 14 in]
      }
      frame "Data: CreatDataFolder" {
        # "Do not put any code in this frame.\n(It is a separator no-op. You can make a copy of this frame to create a new Data frame)"
        n341 = call "DataRootPathFGV.vi"("Error In"=w897, "action (write)"=enum16{"write", "read"}."read") -> ("Error Out"=w905:errorcluster, "PathOut"=w908:path)  [unwired: 8 in]
        n342 = Build Path(base path=w908, name or relative path="3DScanData") -> (appended path=w906:path)
        n343 = call <vilib>:"Check if File or Folder Exists.vi"("error in (no error)"=w905, "path"=w906) -> ("error out"=w899:errorcluster, "file or folder exists?"=w904:bool, "dup path"=w901:path)  [unwired: 7 in]
        n344 = case shown="False" w904 {
          tunnel: w901 -> [w916 w918]
          tunnel: [w914 w918] -> w900
          tunnel: w899 -> [w915 w917]
          tunnel: [w913 w917] -> w898
          frame False {
            # "if folder not exist, creat folder"
            n345 = Create Folder(path (use dialog)=w916, error in=w915) -> (created path=w914:path, error out=w913:errorcluster)  [unwired: 1 in, 1 out]
          }
          frame True {
            # "If folder exist, do nothing"
          }
        }
        n346 = Bundle By Name(cluster=w903, "SaveFilePath"=w900) -> (w902:T15)
        n347 = call <vilib>:"Add State(s) to Queue__JKI_lib_State_Machine.vi"("State(s) in (\"\")"=w912) -> ("States Out"=w911:string)  [unwired: 14 in]
      }
      frame "---------- UI ----------" {
        # "Do not put any code in this frame.\n(It is a separator no-op. You can make a copy of this frame to create a new UI frame)"
        n348 = call <vilib>:"Add State(s) to Queue__JKI_lib_State_Machine.vi"("State(s) in (\"\")"=w923) -> ("States Out"=w922:string)  [unwired: 14 in]
      }
      frame "UI: ReadyToSave" {
        # "Do not put any code in this frame.\n(It is a separator no-op. You can make a copy of this frame to create a new UI frame)"
        n349 = property on="Save Button" class="Bool"("DisabledEnum"=T6."Enabled" ("Disabled")) -> ()  [unwired: 2 in, 2 out]
        n350 = call <vilib>:"Add State(s) to Queue__JKI_lib_State_Machine.vi"("State(s) in (\"\")"=w929) -> ("States Out"=w928:string)  [unwired: 14 in]
      }
      frame "UI: StartUp" {
        w930 = T6."Disabled and Grayed Out" ("Disabled")
        # "Do not put any code in this frame.\n(It is a separator no-op. You can make a copy of this frame to create a new UI frame)"
        n351 = property on="Stage COM port" class="VISAName"("DisabledEnum"=w930) -> ()  [unwired: 2 in, 2 out]
        n352 = property on="Range Finder COM" class="VISAName"("DisabledEnum"=w930) -> ()  [unwired: 2 in, 2 out]
        n353 = property on="3DProfileScan" class="Bool"("DisabledEnum"=w930) -> ()  [unwired: 2 in, 2 out]
        n354 = property on="Plot 3D" class="Bool"("DisabledEnum"=w930) -> ()  [unwired: 2 in, 2 out]
        n355 = property on="Remove Z outlier" class="Bool"("DisabledEnum"=w930) -> ()  [unwired: 2 in, 2 out]
        n356 = property on="Interpolate Scan" class="Bool"("DisabledEnum"=w930) -> ()  [unwired: 2 in, 2 out]
        n357 = property on="Save Button" class="Bool"("DisabledEnum"=w930) -> ()  [unwired: 2 in, 2 out]
        n358 = local write "Tab Control"(T2."Stage Setting" ("Tab Control")) -> ()
        n359 = property on="Calc follow scan" class="Bool"("DisabledEnum"=w930) -> ()  [unwired: 2 in, 2 out]
        n360 = property on="Follow Scan" class="Bool"("DisabledEnum"=w930) -> ()  [unwired: 2 in, 2 out]
        n361 = property on="ParseLocationData" class="Bool"("DisabledEnum"=w930) -> ()  [unwired: 2 in, 2 out]
        n362 = property on="X-Axis configuration" class="Clust (strict)"("DisabledEnum"=w930) -> ()  [unwired: 2 in, 2 out]
        n363 = property on="Y-Axis configuration" class="Clust (strict)"("DisabledEnum"=w930) -> ()  [unwired: 2 in, 2 out]
        n364 = property on="Z-Axis configuration" class="Clust (strict)"("DisabledEnum"=w930) -> ()  [unwired: 2 in, 2 out]
        n365 = property on="Set Origin" class="Bool"("DisabledEnum"=w930) -> ()  [unwired: 2 in, 2 out]
        n366 = property on="Poll grbl position?" class="Bool (strict)"("DisabledEnum"=w930) -> ()  [unwired: 2 in, 2 out]
        n367 = property on="X++" class="Bool"("DisabledEnum"=w930) -> ()  [unwired: 2 in, 2 out]
        n368 = property on="X--" class="Bool"("DisabledEnum"=w930) -> ()  [unwired: 2 in, 2 out]
        n369 = property on="Y++" class="Bool"("DisabledEnum"=w930) -> ()  [unwired: 2 in, 2 out]
        n370 = property on="Y--" class="Bool"("DisabledEnum"=w930) -> ()  [unwired: 2 in, 2 out]
        n371 = property on="Z++" class="Bool"("DisabledEnum"=w930) -> ()  [unwired: 2 in, 2 out]
        n372 = property on="Z--" class="Bool"("DisabledEnum"=w930) -> ()  [unwired: 2 in, 2 out]
        n373 = property on="Hault" class="Bool"("DisabledEnum"=w930) -> ()  [unwired: 2 in, 2 out]
        n374 = property on="GoToZero" class="Bool"("DisabledEnum"=w930) -> ()  [unwired: 2 in, 2 out]
        n375 = property on="Home" class="Bool"("DisabledEnum"=w930) -> ()  [unwired: 2 in, 2 out]
        n376 = call <vilib>:"Add State(s) to Queue__JKI_lib_State_Machine.vi"("State(s) in (\"\")"=w936) -> ("States Out"=w935:string)  [unwired: 14 in]
      }
      frame "UI: FollowScanDone" {
        # "Do not put any code in this frame.\n(It is a separator no-op. You can make a copy of this frame to create a new UI frame)"
        n377 = property on="ParseLocationData" class="Bool"("DisabledEnum"=T6."Enabled" ("Disabled")) -> ()  [unwired: 2 in, 2 out]
        n378 = call <vilib>:"Add State(s) to Queue__JKI_lib_State_Machine.vi"("State(s) in (\"\")"=w942) -> ("States Out"=w941:string)  [unwired: 14 in]
      }
      frame "UI: 3DScanDone" {
        w943 = T6."Disabled and Grayed Out" ("Disabled")
        # "Do not put any code in this frame.\n(It is a separator no-op. You can make a copy of this frame to create a new UI frame)"
        n379 = property on="Interpolate Scan" class="Bool"("DisabledEnum"=w943) -> ()  [unwired: 2 in, 2 out]
        n380 = property on="Follow Scan" class="Bool"("DisabledEnum"=w943) -> ()  [unwired: 2 in, 2 out]
        n381 = property on="ParseLocationData" class="Bool"("DisabledEnum"=w943) -> ()  [unwired: 2 in, 2 out]
        n382 = property on="Plot 3D" class="Bool"("DisabledEnum"=T6."Enabled" ("Disabled")) -> ()  [unwired: 2 in, 2 out]
        n383 = property on="Calc follow scan" class="Bool"("DisabledEnum"=w943) -> ()  [unwired: 2 in, 2 out]
        n384 = property on="Remove Z outlier" class="Bool"("DisabledEnum"=w943) -> ()  [unwired: 2 in, 2 out]
        n385 = call <vilib>:"Add State(s) to Queue__JKI_lib_State_Machine.vi"("State(s) in (\"\")"=w949) -> ("States Out"=w948:string)  [unwired: 14 in]
      }
      frame "UI: Exit" {
        w950 = T6."Enabled" ("Disabled")
        # "Do not put any code in this frame.\n(It is a separator no-op. You can make a copy of this frame to create a new UI frame)"
        n386 = property on="Stage COM port" class="VISAName"("DisabledEnum"=w950) -> ()  [unwired: 2 in, 2 out]
        n387 = property on="Range Finder COM" class="VISAName"("DisabledEnum"=w950) -> ()  [unwired: 2 in, 2 out]
        n388 = property on="X-Axis configuration" class="Clust (strict)"("DisabledEnum"=w950) -> ()  [unwired: 2 in, 2 out]
        n389 = property on="Y-Axis configuration" class="Clust (strict)"("DisabledEnum"=w950) -> ()  [unwired: 2 in, 2 out]
        n390 = property on="Z-Axis configuration" class="Clust (strict)"("DisabledEnum"=w950) -> ()  [unwired: 2 in, 2 out]
        n391 = call <vilib>:"Add State(s) to Queue__JKI_lib_State_Machine.vi"("State(s) in (\"\")"=w955) -> ("States Out"=w954:string)  [unwired: 14 in]
      }
      frame "UI: SysReady" {
        # "System finished start up and ready for use\n(It is a separator no-op. You can make a copy of this frame to create a new UI frame)"
        n392 = call <vilib>:"Add State(s) to Queue__JKI_lib_State_Machine.vi"("State(s) in (\"\")"=w960) -> ("States Out"=w959:string)  [unwired: 14 in]
      }
      frame "UI: Update" {
        # "Do not put any code in this frame.\n(It is a separator no-op. You can make a copy of this frame to create a new UI frame)"
        n393 = Unbundle By Name(w965) -> ("Sys Status"=w963:T1, "StageHomed?"=w961:bool)
        "Sys Status" <- w963
        n394 = Unbundle By Name(w963) -> ("Stage"=w962:bool)
        n395 = case shown="True" w961 {
          frame False {
          }
          frame True {
            w969 = T6."Enabled" ("Disabled")
            n396 = property on="GoToZero" class="Bool"("DisabledEnum"=w969) -> ()  [unwired: 2 in, 2 out]
            n397 = property on="3DProfileScan" class="Bool"("DisabledEnum"=w969) -> ()  [unwired: 2 in, 2 out]
          }
        }
        n398 = case shown="True" w962 {
          frame False {
          }
          frame True {
            w970 = T6."Enabled" ("Disabled")
            n399 = property on="Set Origin" class="Bool"("DisabledEnum"=w970) -> ()  [unwired: 2 in, 2 out]
            n400 = property on="Poll grbl position?" class="Bool (strict)"("DisabledEnum"=w970) -> ()  [unwired: 2 in, 2 out]
            n401 = property on="X++" class="Bool"("DisabledEnum"=w970) -> ()  [unwired: 2 in, 2 out]
            n402 = property on="X--" class="Bool"("DisabledEnum"=w970) -> ()  [unwired: 2 in, 2 out]
            n403 = property on="Y++" class="Bool"("DisabledEnum"=w970) -> ()  [unwired: 2 in, 2 out]
            n404 = property on="Y--" class="Bool"("DisabledEnum"=w970) -> ()  [unwired: 2 in, 2 out]
            n405 = property on="Z++" class="Bool"("DisabledEnum"=w970) -> ()  [unwired: 2 in, 2 out]
            n406 = property on="Z--" class="Bool"("DisabledEnum"=w970) -> ()  [unwired: 2 in, 2 out]
            n407 = property on="Hault" class="Bool"("DisabledEnum"=w970) -> ()  [unwired: 2 in, 2 out]
            n408 = property on="Home" class="Bool"("DisabledEnum"=w970) -> ()  [unwired: 2 in, 2 out]
          }
        }
        n409 = call <vilib>:"Add State(s) to Queue__JKI_lib_State_Machine.vi"("State(s) in (\"\")"=w968) -> ("States Out"=w967:string)  [unwired: 14 in]
      }
      frame "UI: Initialize" {
        # "Initialize the User Interface, here.\n(this is called automatically, by the Macro: Init)"
        n410 = call <vilib>:"Add State(s) to Queue__JKI_lib_State_Machine.vi"("State(s) in (\"\")"=w975) -> ("States Out"=w974:string)  [unwired: 14 in]
      }
      frame "UI: Cursor Set" {
        # "Argument"
        # "Set and Unset Cursor Busy.\n(Usage: \"UI: Cursor Set >> Busy|Idle\")"
        n411 = case shown="\"Idle\", Default" w977 {
          tunnel: w979 -> [w984 w986]
          tunnel: [w983 w985] -> w978
          frame "Idle", Default {
            n412 = call <vilib>:"Unset Busy.vi"("error in (no error)"=w984) -> ("error out"=w983:errorcluster)  [unwired: 10 in]
          }
          frame "Busy" {
            n413 = call <vilib>:"Set Busy.vi"("error in (no error)"=w986) -> ("error out"=w985:errorcluster)  [unwired: 9 in, 1 out]
          }
        }
        n414 = call <vilib>:"Add State(s) to Queue__JKI_lib_State_Machine.vi"("State(s) in (\"\")"=w982) -> ("States Out"=w981:string)  [unwired: 14 in]
      }
      frame "UI: Front Panel State" {
        # "Argument"
        # "Set Front Panel Open or Closed\n(Usage: \"UI: Front Panel State >> Open|Close\")"
        n415 = Unbundle By Name(w990) -> ("Core.Current VI Reference"=w989:refnum<vi>)
        n416 = case shown="\"Open\", \"Standard\", Default" w988 {
          tunnel: w992 -> [w1000 w1015 w1026 w1039 w1052]
          tunnel: [w1002 w1016 w1028 w1041 w1054] -> w991
          tunnel: w989 -> [w1001 w1013 w1027 w1040 w1053]
          frame "Open", "Standard", Default {
            w995 = T10."Standard" ("State")
            n417 = property class="VI"(reference=w1001, error in=w1000) -> (reference out=w998:refnum<vi>, error out=w999:errorcluster, "FP.State"=w997:T10)
            n418 = Not Equal?(x=w997, y=w995) -> (x != y?=w996:bool)
            n419 = case shown="True" w996 {
              tunnel: [w1006 w1008] -> w1002
              tunnel: w999 -> [w1005 w1008]
              tunnel: w998 -> [w1004 _]
              tunnel: w995 -> [w1003 _]
              frame True {
                n420 = invoke class="VI" method="FP.Open"(reference=w1004, error in=w1005, "Activate"=TRUE, "State"=w1003) -> (error out=w1006:errorcluster)  [unwired: 1 in, 4 out]
              }
              frame False {
              }
            }
          }
          frame "Close", "Closed" {
            n421 = property class="VI"(reference=w1013, error in=w1015) -> (reference out=w1012:refnum<vi>, error out=w1014:errorcluster, "FP.State"=w1010:T10)
            n422 = Not Equal?(x=w1010, y=T10."Closed" ("Front Panel Window:State")) -> (x != y?=w1009:bool)
            n423 = case shown="True" w1009 {
              tunnel: [w1017 w1020] -> w1016
              tunnel: w1014 -> [w1017 w1019]
              tunnel: w1012 -> [_ w1018]
              frame False {
              }
              frame True {
                n424 = invoke class="VI" method="FP.Close"(reference=w1018, error in=w1019) -> (error out=w1020:errorcluster)  [unwired: 1 in, 2 out]
              }
            }
          }
          frame "Hidden", "Hide" {
            w1021 = T10."Hidden" ("State")
            n425 = property class="VI"(reference=w1027, error in=w1026) -> (reference out=w1024:refnum<vi>, error out=w1025:errorcluster, "FP.State"=w1023:T10)
            n426 = Not Equal?(x=w1023, y=w1021) -> (x != y?=w1022:bool)
            n427 = case shown="True" w1022 {
              tunnel: [w1032 w1033] -> w1028
              tunnel: w1025 -> [w1031 w1033]
              tunnel: w1024 -> [w1030 _]
              tunnel: w1021 -> [w1029 _]
              frame True {
                n428 = invoke class="VI" method="FP.Open"(reference=w1030, error in=w1031, "State"=w1029) -> (error out=w1032:errorcluster)  [unwired: 2 in, 4 out]
              }
              frame False {
              }
            }
          }
          frame "Minimize", "Minimized" {
            w1034 = T10."Minimized" ("State")
            n429 = property class="VI"(reference=w1040, error in=w1039) -> (reference out=w1037:refnum<vi>, error out=w1038:errorcluster, "FP.State"=w1036:T10)
            n430 = Not Equal?(x=w1036, y=w1034) -> (x != y?=w1035:bool)
            n431 = case shown="True" w1035 {
              tunnel: [w1045 w1046] -> w1041
              tunnel: w1038 -> [w1044 w1046]
              tunnel: w1037 -> [w1043 _]
              tunnel: w1034 -> [w1042 _]
              frame True {
                n432 = invoke class="VI" method="FP.Open"(reference=w1043, error in=w1044, "State"=w1042) -> (error out=w1045:errorcluster)  [unwired: 2 in, 4 out]
              }
              frame False {
              }
            }
          }
          frame "Maximize", "Maximized" {
            w1047 = T10."Maximized" ("State")
            n433 = property class="VI"(reference=w1053, error in=w1052) -> (reference out=w1050:refnum<vi>, error out=w1051:errorcluster, "FP.State"=w1049:T10)
            n434 = Not Equal?(x=w1049, y=w1047) -> (x != y?=w1048:bool)
            n435 = case shown="True" w1048 {
              tunnel: [w1058 w1059] -> w1054
              tunnel: w1051 -> [w1057 w1059]
              tunnel: w1050 -> [w1056 _]
              tunnel: w1047 -> [w1055 _]
              frame True {
                n436 = invoke class="VI" method="FP.Open"(reference=w1056, error in=w1057, "State"=w1055) -> (error out=w1058:errorcluster)  [unwired: 2 in, 4 out]
              }
              frame False {
              }
            }
          }
        }
        n437 = call <vilib>:"Add State(s) to Queue__JKI_lib_State_Machine.vi"("State(s) in (\"\")"=w994) -> ("States Out"=w993:string)  [unwired: 14 in]
      }
      frame "---------- Stage ----------" {
        # "Template Separator\n(You can make a copy of, or modify, this frame)"
        n438 = call <vilib>:"Add State(s) to Queue__JKI_lib_State_Machine.vi"("State(s) in (\"\")"=w1064) -> ("States Out"=w1063:string)  [unwired: 14 in]
      }
      frame "Stage: Initialize" {
        # "Initialize stage controler\n(Open connection and check)"
        n439 = call "Initialize Serial Port.vi"("VISA resource name"="Stage COM port", "baud rate (115200)"=u32 115200, "error in (no error)"=w1074) -> ("error out"=w1071:errorcluster)  [unwired: 12 in]
        n440 = call "Get Version.vi"("error in (no error)"=w1071) -> ("Version information"=→"Version information":string, "error out"=w1065:errorcluster)  [unwired: 12 in, 1 out]
        n441 = case shown="No Error" w1065 {
          selector: w1065 -> [w1077 _]
          tunnel: [w1077 w1078] -> w1070
          frame No Error {
          }
          frame Error {
            # "If grbl respond is wrong"
            n442 = xnode "Error Ring"() -> ("error out"=w1078:errorcluster)
          }
        }
        n443 = case shown="No Error" w1065 {
          tunnel: [w1086 w1088] -> w1073
          tunnel: w1066 -> [w1085 w1088]
          tunnel: "Stage COM port" -> [w1084 _]
          frame No Error {
            n444 = Bundle By Name(cluster=w1085, "Sys Status.Stage"=TRUE, "StageCOM"=w1084) -> (w1086:T15)
          }
          frame Error {
          }
        }
        n445 = call <vilib>:"Add State(s) to Queue__JKI_lib_State_Machine.vi"("State(s) in (\"\")"=w1076) -> ("States Out"=w1075:string)  [unwired: 14 in]
      }
      frame "Stage: Reset" {
        # "Reset grbl\n(Ctrl+x)"
        n446 = call "Reset.vi"("error in (no error)"=w1090) -> ("error out"=w1091:errorcluster)  [unwired: 14 in]
        n447 = call <vilib>:"Add State(s) to Queue__JKI_lib_State_Machine.vi"("State(s) in (\"\")"=w1094) -> ("States Out"=w1093:string)  [unwired: 14 in]
      }
      frame "Stage: Config" {
        # "set G code parser and default speed 2000"
        # "Initialize stage controler and set default configuration\n()"
        n448 = call "Config IO.vi"("Pulse time us"=u32 3, "Soft limit enable"=TRUE, "Hard limit enable"=TRUE, "Step idle delay ms (255 keep)"=u8 25, "Step pulse invert"=T14 {"Reverse X"=FALSE, "Reverse Y"=FALSE, "Reverse Z"=FALSE}, "Axis direction"=T14 {"Reverse X"=TRUE, "Reverse Y"=TRUE, "Reverse Z"=TRUE}, "error in (no error)"=w1105, "Pins direction"=T13 {"Invert enable pin"=FALSE, "Invert limit pin"=FALSE, "Invert probe pin"=FALSE}) -> ("error out"=w1123:errorcluster)  [unwired: 7 in]
        n449 = call "Config Axis.vi"("X-Axis configuration"="X-Axis configuration", "Y-Axis configuration"="Y-Axis configuration", "Z-Axis configuration"="Z-Axis configuration", "error in (no error)"=w1123) -> ("error out"=w1122:errorcluster)  [unwired: 11 in]
        n450 = call "Config Home.vi"("Homing direction invert"=T14 {"Reverse X"=TRUE, "Reverse Y"=TRUE, "Reverse Z"=TRUE}, "Homing cycle enable"=TRUE, "Homing locate feed rate\tmm/min"=u32 100 ("Homing locate feed rate\tmm/min"), "Homing search seek rate\tmm/min"=u32 3000 ("Homing search seek rate\tmm/min"), "Homing switch debounce delay\tms"=u32 25 ("Homing switch debounce delay\tms"), "error in (no error)"=w1122, "Homing switch pull-off distance\tmm"=u32 2 ("Homing switch pull-off distance\tmm")) -> ("error out"=w1121:errorcluster)  [unwired: 8 in]
        n451 = call "Release Lock from Alarm.vi"("error in (no error)"=w1121) -> ("error out"=w1120:errorcluster)  [unwired: 14 in]
        n452 = call "Get Configuration.vi"("error in (no error)"=w1120) -> ("Config"=→"Current Config":string, "error out"=w1101:errorcluster)  [unwired: 13 in]
        n453 = Concatenate Strings("G1F2000" ("Data to write"), "\r") -> (w1097:string)
        n454 = call "Send-Receive Serial Port.vi"("Data to write"=w1097, "error in (no error)"=w1101) -> ("error out"=w1100:errorcluster)  [unwired: 12 in, 1 out]
        n455 = call <vilib>:"Add State(s) to Queue__JKI_lib_State_Machine.vi"("State(s) in (\"\")"=w1125) -> ("States Out"=w1124:string)  [unwired: 14 in]
      }
      frame "Stage: Home" {
        # "Home Stage\n(You can make a copy of, or modify, this frame)"
        n456 = Two Button Dialog(message="Stage will home, please retrack fiber probe and make sure no object is in its way!", 1:"Cancel" ("F button name (\"Cancel\")"), 2:"Confirm" ("T button name (\"OK\")")) -> (T button?=w1126:bool)
        n457 = case shown="True" w1126 {
          tunnel: [w1140 w1150] -> w1134
          tunnel: [w1139 w1149] -> w1133
          tunnel: w1132 -> [w1139 w1148]
          tunnel: w1130 -> [w1140 w1147]
          frame False {
            n458 = One Button Dialog(message="You must home stage before doing any scanning! Some function of the program is now disabled!", button name ("OK")="Confirm") -> ()  [unwired: 1 out]
          }
          frame True {
            # "Update origin"
            n459 = call <vilib>:"Set Busy.vi"("error in (no error)"=w1147) -> ("error out"=w1142:errorcluster)  [unwired: 9 in, 1 out]
            n460 = call "Go home.vi"("Maximum wait time (45sec)"=30, "error in (no error)"=w1142) -> ("error out"=w1146:errorcluster)  [unwired: 13 in]
            n461 = call <vilib>:"Unset Busy.vi"("error in (no error)"=w1146) -> ("error out"=w1141:errorcluster)  [unwired: 10 in]
            n462 = Unbundle By Name(w1146) -> ("status"=w1145:bool)
            n463 = call "Get Status.vi"("error in (no error)"=w1141) -> ("Current position"=w1143:cluster{"X":sgl, "Y":sgl, "Z":sgl}, "error out"=w1150:errorcluster)  [unwired: 10 in, 3 out]
            "Stage Home MPos" <- w1143
            n464 = Not(x=w1145) -> (.not. x?=w1144:bool)
            n465 = local write "Current Machine Pos"(w1143) -> ()
            n466 = Bundle By Name(cluster=w1148, "StageHomed?"=w1144, "HomeMposOrigin"=w1143) -> (w1149:T15)
          }
        }
        n467 = call <vilib>:"Add State(s) to Queue__JKI_lib_State_Machine.vi"("State(s) in (\"\")"=w1136) -> ("States Out"=w1135:string)  [unwired: 14 in]
      }
      frame "Stage: GoToZero" {
        # "Go to scanning origin marked on the platform\n(Go to scanning start and set original position)"
        n468 = Unbundle By Name(w1153) -> ("StageHomed?"=w1152:bool)
        n469 = case shown="True" w1152 {
          tunnel: w1157 -> [w1163 w1174]
          tunnel: [w1163 w1173] -> w1156
          tunnel: [w1162 w1172] -> w1155
          tunnel: w1153 -> [w1162 w1171]
          frame False {
            # "stage not homed, do nothing"
            n470 = One Button Dialog(message="Stage not homed! Could not go to scan origin marked on stage platform! Please home stage and go to scan origin manually using the stage control.", button name ("OK")="Confirm") -> ()  [unwired: 1 out]
          }
          frame True {
            # "reset encoder"
            # "If stage is homed, move to scan origin"
            n471 = stacked-sequence {
              seq-local: [w1180 _] -> [_ w1195]
              tunnel: w1174 -> [w1181 _]
              tunnel: [_ w1194] -> w1164
              frame #0 {
                # "Move laterally"
                n472 = call "Get Status.vi"("error in (no error)"=w1181) -> ("Status"=w1179:T9, "Current position"=w1175:cluster{"X":sgl, "Y":sgl, "Z":sgl}, "error out"=w1176:errorcluster)  [unwired: 10 in, 2 out]
                n473 = Equal?(x=Status."Idle" ("Status"), y=w1179) -> (x = y?=w1177:bool)
                n474 = case shown="True" w1177 {
                  tunnel: w1176 -> [w1183 w1193]
                  tunnel: [w1183 w1186] -> w1180
                  tunnel: w1175 -> [_ w1185]
                  frame False {
                    n475 = One Button Dialog(message="Could not go to starting point. ") -> ()  [unwired: 1 in, 1 out]
                  }
                  frame True {
                    n476 = Unbundle By Name(w1185) -> ("Z"=w1184:sgl)
                    n477 = call <vilib>:"Set Busy.vi"("error in (no error)"=w1193) -> ("error out"=w1187:errorcluster)  [unwired: 9 in, 1 out]
                    n478 = call "Go to Position.vi"("X (mm)"=sgl 23.0, "Speed (2000 mm/min)"=sgl 3000.0 ("Speed (mm/min)"), "Overwright speed? (F)"=TRUE, "Y (mm)"=sgl 72.0, "Z (mm)"=w1184, "error in (no error)"=w1187) -> ("error out"=w1190:errorcluster)  [unwired: 9 in]
                    n479 = call <vilib>:"Unset Busy.vi"("error in (no error)"=w1190) -> ("error out"=w1186:errorcluster)  [unwired: 10 in]
                  }
                }
              }
              frame #1 {
                # "Go down to 0"
                n480 = call "Get Status.vi"("error in (no error)"=w1195) -> ("Status"=w1199:T9, "error out"=w1196:errorcluster)  [unwired: 10 in, 3 out]
                n481 = Equal?(x=Status."Idle" ("Status"), y=w1199) -> (x = y?=w1197:bool)
                n482 = case shown="True" w1197 {
                  tunnel: w1196 -> [w1201 w1210]
                  tunnel: [w1201 w1203] -> w1194
                  frame False {
                    n483 = One Button Dialog(message="Could not go to starting point. ") -> ()  [unwired: 1 in, 1 out]
                  }
                  frame True {
                    n484 = call <vilib>:"Set Busy.vi"("error in (no error)"=w1210) -> ("error out"=w1204:errorcluster)  [unwired: 9 in, 1 out]
                    n485 = call "Go to Position.vi"("X (mm)"=sgl 23.0, "Speed (2000 mm/min)"=sgl 3000.0 ("Speed (mm/min)"), "Overwright speed? (F)"=TRUE, "Y (mm)"=sgl 72.0, "Z (mm)"=sgl 0.0, "error in (no error)"=w1204) -> ("error out"=w1207:errorcluster)  [unwired: 9 in]
                    n486 = call <vilib>:"Unset Busy.vi"("error in (no error)"=w1207) -> ("error out"=w1203:errorcluster)  [unwired: 10 in]
                  }
                }
              }
            }
            n487 = call "Get Status.vi"("error in (no error)"=w1164) -> ("Current position"=w1165:cluster{"X":sgl, "Y":sgl, "Z":sgl}, "error out"=w1166:errorcluster)  [unwired: 10 in, 3 out]
            n488 = Bundle By Name(cluster=w1171, "ScanOrigin"=w1165) -> (w1172:T15)
            n489 = call "LabJack_FGV_T4.vi"("Operation(Read)"=enum16{"Write", "Read"}."Read" ("Operation"), "error in (no error)"=w1166) -> ("error out"=w1169:errorcluster, "Read data"=w1168:i32)  [unwired: 8 in]
            n490 = call "LJM_eReadName.vi"("Handle In"=w1168, "Name"="DIO4_EF_READ_A_AND_RESET", "error in"=w1169) -> ("error out"=w1173:errorcluster)  [unwired: 10 in, 2 out]
            n491 = local write "Scan Origin MPos"(w1165) -> ()
          }
        }
        n492 = call <vilib>:"Add State(s) to Queue__JKI_lib_State_Machine.vi"("State(s) in (\"\")"=w1159) -> ("States Out"=w1158:string)  [unwired: 14 in]
      }
      frame "Stage: RaiseFiber" {
        # "Template Separator\n(You can make a copy of, or modify, this frame)"
        n493 = call "Get Status.vi"("error in (no error)"=w1211) -> ("Status"=w1220:T9, "Current position"=w1216:cluster{"X":sgl, "Y":sgl, "Z":sgl}, "error out"=w1217:errorcluster)  [unwired: 10 in, 2 out]
        n494 = Equal?(x=Status."Idle" ("Status"), y=w1220) -> (x = y?=w1218:bool)
        n495 = Unbundle By Name(w1216) -> ("X"=w1215:sgl, "Y"=w1214:sgl, "Z"=w1213:sgl)
        n496 = case shown="True" w1218 {
          tunnel: w1217 -> [w1226 w1237]
          tunnel: [w1226 w1232] -> w1212
          tunnel: w1215 -> [_ w1231]
          tunnel: w1214 -> [_ w1230]
          tunnel: w1213 -> [_ w1229]
          frame False {
            n497 = One Button Dialog(message="Could not go to starting point. ") -> ()  [unwired: 1 in, 1 out]
          }
          frame True {
            n498 = call <vilib>:"Set Busy.vi"("error in (no error)"=w1237) -> ("error out"=w1233:errorcluster)  [unwired: 9 in, 1 out]
            n499 = Add(x=w1229, y=sgl 20.0) -> (x+y=w1227:sgl)
            n500 = call "Go to Position.vi"("X (mm)"=w1231, "Speed (2000 mm/min)"=sgl 3000.0 ("Speed (mm/min)"), "Overwright speed? (F)"=TRUE, "Y (mm)"=w1230, "Z (mm)"=w1227, "error in (no error)"=w1233) -> ("error out"=w1236:errorcluster)  [unwired: 9 in]
            n501 = call <vilib>:"Unset Busy.vi"("error in (no error)"=w1236) -> ("error out"=w1232:errorcluster)  [unwired: 10 in]
          }
        }
        n502 = call <vilib>:"Add State(s) to Queue__JKI_lib_State_Machine.vi"("State(s) in (\"\")"=w1224) -> ("States Out"=w1223:string)  [unwired: 14 in]
      }
      frame "Stage: SendCommand" {
        # "Template Separator\n(You can make a copy of, or modify, this frame)"
        n503 = call "Send-Receive Serial Port.vi"("Data to write"=w1239, "error in (no error)"=w1240) -> ("error out"=w1241:errorcluster)  [unwired: 12 in, 1 out]
        n504 = call <vilib>:"Add State(s) to Queue__JKI_lib_State_Machine.vi"("State(s) in (\"\")"=w1244) -> ("States Out"=w1243:string)  [unwired: 14 in]
      }
      frame "Stage: Close" {
        # "Close Stage connection\n(You can make a copy of, or modify, this frame)"
        n505 = Unbundle By Name(w1246) -> ("Sys Status.Stage"=w1248:bool)
        n506 = case shown="True" w1248 {
          tunnel: [w1254 w1259] -> w1250
          tunnel: w1249 -> [w1254 w1258]
          tunnel: w1246 -> [w1253 w1257]
          tunnel: [w1253 w1255] -> w1247
          frame False {
          }
          frame True {
            n507 = Bundle By Name(cluster=w1257, "Sys Status.Stage"=FALSE ("Sys Status.Stage COM")) -> (w1255:T15)
            n508 = call "Close Serial Port.vi"("error in (no error)"=w1258) -> ("error out"=w1259:errorcluster)  [unwired: 14 in]
          }
        }
        n509 = call <vilib>:"Add State(s) to Queue__JKI_lib_State_Machine.vi"("State(s) in (\"\")"=w1252) -> ("States Out"=w1251:string)  [unwired: 14 in]
      }
      frame "---------- AccuRange ----------" {
        # "Template Separator\n(You can make a copy of, or modify, this frame)"
        n510 = call <vilib>:"Add State(s) to Queue__JKI_lib_State_Machine.vi"("State(s) in (\"\")"=w1264) -> ("States Out"=w1263:string)  [unwired: 14 in]
      }
      frame "AccuRange: Initialize" {
        w1277 = u16 0 items=["None", "XON/XOFF", "RTS/CTS", "XON/XOFF & RTS/CTS", "DTR/DSR", "XON/XOFF & DTR/DSR"] ("flow control (0:none)")
        # "clear VISA buffer"
        # "Open AccuRange COM port\n(You can make a copy of, or modify, this frame)"
        n511 = call-poly "VISA Configure Serial Port"("VISA resource name"="Range Finder COM", "termination char\n(0xA = '\\n' = LF)"=u8 255 ("termination char\n(0xA = '\\n' = LF)"), "Enable Termination\nChar (T)"=TRUE ("Enable Termination\nChar (T)"), "baud rate (9600)"=u32 115200, "error in (no error)"=w1276, "flow control (0:none)"=w1277) -> ("VISA resource name out"=w1272:refnum<visa-resource-name>, "error out"=w1270:errorcluster)  [unwired: 8 in]
        n512 = VISA Clear(VISA resource name=w1272, error in (no error)=w1270) -> (VISA resource name out=w1271:refnum<visa-resource-name>, error out=w1269:errorcluster)
        n513 = case shown="Error" w1269 {
          selector: w1269 -> [w1281 _]
          tunnel: w1271 -> [w1284 _]
          tunnel: w1274 -> [w1283 w1287]
          tunnel: [w1282 w1287] -> w1273
          tunnel: [w1281 w1286] -> w1265
          frame No Error {
            n514 = Bundle By Name(cluster=w1283, "RangeCOM"=w1284, "Sys Status.RangerFinder"=TRUE) -> (w1282:T15)
          }
          frame Error {
            n515 = xnode "Error Ring"() -> ("error out"=w1286:errorcluster)
          }
        }
        n516 = call <vilib>:"Add State(s) to Queue__JKI_lib_State_Machine.vi"("State(s) in (\"\")"=w1280) -> ("States Out"=w1279:string)  [unwired: 14 in]
      }
      frame "AccuRange: Config" {
        # "Config range finder\n(You can make a copy of, or modify, this frame)"
        n517 = Unbundle By Name(w1310) -> ("RangeCOM"=w1296:refnum<visa-resource-name>)
        n518 = VISA Write(VISA resource name=w1296, write buffer="S80.X5.", error in (no error)=w1295) -> (VISA resource name out=w1309:refnum<visa-resource-name>, error out=w1300:errorcluster)  [unwired: 1 out]
        n519 = VISA Write(VISA resource name=w1309, write buffer="N.", error in (no error)=w1300) -> (VISA resource name out=w1301:refnum<visa-resource-name>, error out=w1299:errorcluster)  [unwired: 1 out]
        n520 = VISA Write(VISA resource name=w1301, write buffer="L1.", error in (no error)=w1299) -> (VISA resource name out=w1302:refnum<visa-resource-name>, error out=w1298:errorcluster)  [unwired: 1 out]
        n521 = VISA Write(VISA resource name=w1302, write buffer="A2.", error in (no error)=w1298) -> (VISA resource name out=w1303:refnum<visa-resource-name>, error out=w1297:errorcluster)  [unwired: 1 out]
        n522 = VISA Write(VISA resource name=w1303, write buffer="P1.", error in (no error)=w1297) -> (error out=w1294:errorcluster)  [unwired: 2 out]
        n523 = call <vilib>:"Add State(s) to Queue__JKI_lib_State_Machine.vi"("State(s) in (\"\")"=w1312) -> ("States Out"=w1311:string)  [unwired: 14 in]
      }
      frame "AccuRange: Start" {
        # "6"
        # "5"
        # "4"
        # "3"
        # "2"
        # "1"
        # "1. Start measurement\n2. Stop data streaming\n3. Flush read buffer to sync\n4. Restart streaming\n5. Set ranger finder loop stop flag\n6. Send user event to start loop"
        # "Start range finder\n(You can make a copy of, or modify, this frame)"
        n524 = Unbundle By Name(w1333) -> ("RangeCOM"=w1327:refnum<visa-resource-name>)
        n525 = Build Array(u8 19) -> (w1324:u8[])
        n526 = Byte Array To String(unsigned byte array=w1324) -> (string=w1321:string)
        n527 = Build Array(u8 17) -> (w1320:u8[])
        n528 = VISA Write(VISA resource name=w1327, write buffer="H1.", error in (no error)=w1326) -> (VISA resource name out=w1322:refnum<visa-resource-name>, error out=w1330:errorcluster)  [unwired: 1 out]
        n529 = Byte Array To String(unsigned byte array=w1320) -> (string=w1317:string)
        n530 = VISA Write(VISA resource name=w1322, write buffer=w1321, error in (no error)=w1330) -> (VISA resource name out=w1315:refnum<visa-resource-name>, error out=w1323:errorcluster)  [unwired: 1 out]
        n531 = VISA Flush I/O Buffer(VISA resource name=w1315, error in (no error)=w1323) -> (VISA resource name out=w1314:refnum<visa-resource-name>, error out=w1316:errorcluster)  [unwired: 1 in]
        n532 = VISA Write(VISA resource name=w1314, write buffer=w1317, error in (no error)=w1316) -> (error out=w1318:errorcluster)  [unwired: 2 out]
        n533 = flat-sequence {
          tunnel: w1318 -> [w1337]
          tunnel: [w1337] -> w1329
          frame #0 {
            n534 = local write "AccuRangeLoopStopFlag"(FALSE ("Stop Read")) -> ()
          }
        }
        n535 = Generate User Event(user event=w1332, event data cluster=TRUE ("event data"), error in=w1329) -> (error out=w1328:errorcluster)  [unwired: 1 in, 1 out]
        n536 = call <vilib>:"Add State(s) to Queue__JKI_lib_State_Machine.vi"("State(s) in (\"\")"=w1336) -> ("States Out"=w1335:string)  [unwired: 14 in]
      }
      frame "AccuRange: Stop" {
        # "stop read before turn off laser ranger. Otherwise cause VISA error and COM port can not be closed."
        # "Stop range finder\n(You can make a copy of, or modify, this frame)"
        n537 = Unbundle By Name(w1347) -> ("RangeCOM"=w1346:refnum<visa-resource-name>, "Sys Status.RangerFinder"=w1340:bool)
        n538 = flat-sequence {
          tunnel: w1345 -> [w1364]
          tunnel: [w1364] -> w1344
          frame #0 {
            n539 = local write "AccuRangeLoopStopFlag"(TRUE ("Stop Read")) -> ()
          }
        }
        n540 = call <userlib>:"Wait (ms)__ogtk.vi"("error in (no error)"=w1344, "milliseconds to wait"=u32 200) -> ("error out"=w1342:errorcluster)  [unwired: 8 in, 1 out]
        n541 = disable-structure shown="Enabled" {
          disable-tunnel: w1346 -> [w1353 _]
          disable-tunnel: [w1352 w1363] -> w1343
          disable-tunnel: w1342 -> [w1351 w1363]
          disable-tunnel: w1340 -> [w1350 _]
          frame Disabled {
            n542 = case shown="True" w1350 {
              tunnel: w1353 -> [_ w1361]
              tunnel: [w1354 w1358] -> w1352
              tunnel: w1351 -> [w1354 w1355]
              frame False {
              }
              frame True {
                n543 = VISA Write(VISA resource name=w1361, write buffer="H2.", error in (no error)=w1355) -> (VISA resource name out=w1360:refnum<visa-resource-name>, error out=w1359:errorcluster)  [unwired: 1 out]
                n544 = call <userlib>:"Wait Until Next ms Multiple__ogtk.vi"("error in (no error)"=w1359, "milliseconds to wait"=u32 500) -> ("error out"=w1357:errorcluster)  [unwired: 8 in, 1 out]
                n545 = VISA Clear(VISA resource name=w1360, error in (no error)=w1357) -> (error out=w1358:errorcluster)  [unwired: 1 out]
              }
            }
          }
          frame Enabled {
          }
        }
        n546 = call <vilib>:"Add State(s) to Queue__JKI_lib_State_Machine.vi"("State(s) in (\"\")"=w1349) -> ("States Out"=w1348:string)  [unwired: 14 in]
      }
      frame "AccuRange: Close" {
        # "Template Separator\n(You can make a copy of, or modify, this frame)"
        n547 = Unbundle By Name(w1367) -> ("RangeCOM"=w1369:refnum<visa-resource-name>, "Sys Status.RangerFinder"=w1372:bool)
        n548 = case shown="True" w1372 {
          tunnel: w1370 -> [w1376 w1378]
          tunnel: [w1376 w1384] -> w1371
          tunnel: w1369 -> [_ w1380]
          tunnel: w1367 -> [w1375 w1383]
          tunnel: [w1375 w1382] -> w1368
          frame False {
            # "If COM is not open, do nothing"
          }
          frame True {
            # "If COM is open, close it"
            n549 = VISA Clear(VISA resource name=w1380, error in (no error)=w1378) -> (VISA resource name out=w1379:refnum<visa-resource-name>, error out=w1377:errorcluster)
            n550 = VISA Close(VISA resource name=w1379, error in (no error)=w1377) -> (error out=w1384:errorcluster)
            n551 = Bundle By Name(cluster=w1383, "Sys Status.RangerFinder"=FALSE) -> (w1382:T15)
          }
        }
        n552 = call <vilib>:"Add State(s) to Queue__JKI_lib_State_Machine.vi"("State(s) in (\"\")"=w1374) -> ("States Out"=w1373:string)  [unwired: 14 in]
      }
      frame "---------- Utility ----------" {
        # "Template Separator\n(You can make a copy of, or modify, this frame)"
        n553 = call <vilib>:"Add State(s) to Queue__JKI_lib_State_Machine.vi"("State(s) in (\"\")"=w1389) -> ("States Out"=w1388:string)  [unwired: 14 in]
      }
      frame "Utility: DestroyQueue" {
        # "Template Separator\n(You can make a copy of, or modify, this frame)"
        n554 = Obtain Queue(name (unnamed)="FLImData", element data type=cluster{"PPIXInt":dbl, "x":dbl} {"PPIXInt"=0.0, "x"=0.0}, error in (no error)=w1391) -> (queue out=w1394:refnum<queue>, error out=w1393:errorcluster)  [unwired: 2 in, 1 out]
        n555 = Release Queue(queue=w1394, error in (no error)=w1393) -> (error out=w1392:errorcluster)  [unwired: 1 in, 2 out]
        n556 = call <vilib>:"Add State(s) to Queue__JKI_lib_State_Machine.vi"("State(s) in (\"\")"=w1399) -> ("States Out"=w1398:string)  [unwired: 14 in]
      }
      frame "Utility: Plot3D" {
        # "Template Separator\n(You can make a copy of, or modify, this frame)"
        n557 = Unbundle By Name(w1405) -> ("3DProfileToPlot"=w1404:cluster{"x(mm)":dbl, "y(mm)":dbl, "z(mm)":dbl}[])
        n558 = for {
          tunnel: w1404 -> [w1413] mode=indexing
          tunnel: [w1412] -> w1403 mode=indexing
          tunnel: [w1411] -> w1402 mode=indexing
          tunnel: [w1410] -> w1401 mode=indexing
          n559 = Unbundle By Name(w1413) -> ("x(mm)"=w1412:dbl, "y(mm)"=w1411:dbl, "z(mm)"=w1410:dbl)
        }
        n560 = call-poly <vilib>:"Plot Helper.vi"("z vector"=w1401, "y vector"=w1402, "x vector"=w1403) -> ("3D Plot lvclass Array out"=→"3D Profile":refnum<class "3D Plot Datatype.lvclass">[])  [unwired: 3 in, 5 out]
        n561 = call <vilib>:"Add State(s) to Queue__JKI_lib_State_Machine.vi"("State(s) in (\"\")"=w1409) -> ("States Out"=w1408:string)  [unwired: 14 in]
      }
      frame "Utility: Dewelling" {
        # "Template Separator\n(e.x. Dewelling >> 1000)"
        n562 = Decimal String To Number(string=w1416) -> (number=w1415:i32)  [unwired: 2 in, 1 out]
        n563 = Wait (ms)(milliseconds to wait=w1415) -> ()  [unwired: 1 out]
        n564 = call <vilib>:"Add State(s) to Queue__JKI_lib_State_Machine.vi"("State(s) in (\"\")"=w1420) -> ("States Out"=w1419:string)  [unwired: 14 in]
      }
      frame "---------- LJT4 ----------" {
        # "Template Separator\n(You can make a copy of, or modify, this frame)"
        n565 = call <vilib>:"Add State(s) to Queue__JKI_lib_State_Machine.vi"("State(s) in (\"\")"=w1425) -> ("States Out"=w1424:string)  [unwired: 14 in]
      }
      frame "LJT4: Initialize" {
        # "Open Connection to T4\n(You can make a copy of, or modify, this frame)"
        n566 = call "LJ_Open.vi"("error in"=w1430, "DeviceType"="LJM_dtT4") -> ("error out"=w1427:errorcluster, "Success?"=w1426:bool, "Handle Out"=w1428:i32)  [unwired: 7 in]
        n567 = call "LabJack_FGV_T4.vi"("Operation(Read)"=enum16{"Write", "Read"}."Write" ("Operation"), "error in (no error)"=w1427, "Write data"=w1428) -> ("error out"=w1434:errorcluster)  [unwired: 7 in, 1 out]
        n568 = Bundle By Name(cluster=w1432, "Sys Status.T4"=w1426) -> (w1433:T15)
        n569 = call <vilib>:"Add State(s) to Queue__JKI_lib_State_Machine.vi"("State(s) in (\"\")"=w1437) -> ("States Out"=w1436:string)  [unwired: 14 in]
      }
      frame "LJT4: RestEncoder" {
        # "Reset encoder \n(by read DIO4_EF_READ_A_AND_RESET)"
        n570 = call "LabJack_FGV_T4.vi"("Operation(Read)"=enum16{"Write", "Read"}."Read" ("Operation"), "error in (no error)"=w1438) -> ("error out"=w1443:errorcluster, "Read data"=w1442:i32)  [unwired: 8 in]
        n571 = call "LJM_eReadName.vi"("Handle In"=w1442, "Name"="DIO4_EF_READ_A_AND_RESET", "error in"=w1443) -> ("error out"=w1439:errorcluster)  [unwired: 10 in, 2 out]
        n572 = call <vilib>:"Add State(s) to Queue__JKI_lib_State_Machine.vi"("State(s) in (\"\")"=w1447) -> ("States Out"=w1446:string)  [unwired: 14 in]
      }
      frame "LJT4: Config" {
        w1452 = 1.0 ("element")
        w1453 = 10.0 ("element")
        w1454 = 0.0 ("element")
        w1456 = "DIO5_EF_ENABLE"
        w1457 = "DIO4_EF_ENABLE"
        # "Config T4 quadrature in\n(You can make a copy of, or modify, this frame)"
        n573 = Build Array(w1457, w1456, "DIO4_EF_INDEX", "DIO5_EF_INDEX", w1457, w1456) -> (w1455:string[])
        n574 = call "LabJack_FGV_T4.vi"("Operation(Read)"=enum16{"Write", "Read"}."Read" ("Operation"), "error in (no error)"=w1449) -> ("error out"=w1461:errorcluster, "Read data"=w1460:i32)  [unwired: 8 in]
        n575 = Build Array(w1454, w1454, w1453, w1453, w1452, w1452) -> (w1451:dbl[])
        n576 = call "LJM_eWriteNames.vi"("Handle In"=w1460, "aNames"=w1455, "aValuesIn"=w1451, "error in"=w1461) -> ("error out"=w1450:errorcluster)  [unwired: 9 in, 2 out]
        n577 = call <vilib>:"Add State(s) to Queue__JKI_lib_State_Machine.vi"("State(s) in (\"\")"=w1465) -> ("States Out"=w1464:string)  [unwired: 14 in]
      }
      frame "LJT4: Close" {
        # "Close T4 conncetion\n(You can make a copy of, or modify, this frame)"
        n578 = Unbundle By Name(w1467) -> ("Sys Status.T4"=w1469:bool)
        n579 = case shown="True" w1469 {
          tunnel: [w1475 w1481] -> w1471
          tunnel: w1470 -> [w1475 w1480]
          tunnel: w1467 -> [w1474 w1478]
          tunnel: [w1474 w1477] -> w1468
          frame False {
          }
          frame True {
            n580 = call "LabJack_FGV_T4.vi"("Operation(Read)"=enum16{"Write", "Read"}."Read" ("Operation"), "error in (no error)"=w1480) -> ("error out"=w1482:errorcluster, "Read data"=w1479:i32)  [unwired: 8 in]
            n581 = call "LJM_Close.vi"("error in"=w1482, "Handle"=w1479) -> ("error out"=w1481:errorcluster)  [unwired: 9 in]
            n582 = Bundle By Name(cluster=w1478, "Sys Status.T4"=FALSE) -> (w1477:T15)
          }
        }
        n583 = call <vilib>:"Add State(s) to Queue__JKI_lib_State_Machine.vi"("State(s) in (\"\")"=w1473) -> ("States Out"=w1472:string)  [unwired: 14 in]
      }
      frame "---------- USBCam ----------" {
        # "Template Separator\n(You can make a copy of, or modify, this frame)"
        n584 = call <vilib>:"Add State(s) to Queue__JKI_lib_State_Machine.vi"("State(s) in (\"\")"=w1488) -> ("States Out"=w1487:string)  [unwired: 14 in]
      }
      frame "USBCam: Initialize" {
        # "Template Separator\n(You can make a copy of, or modify, this frame)"
        n585 = call <vilib>:"IMAQdx Open Camera.vi"("error in"=w1500, "Session In"="CamSession In") -> ("error out"=w1493:errorcluster, "Session Out"=w1495:T4)  [unwired: 1 in, 7 out]
        n586 = call "IMAQ Create"("Image Name"="USB Image", "error in (no error)"=w1500) -> ("New Image"=w1491:T5, "error out"=w1501:errorcluster)  [unwired: 2 in, 1 out]
        "New Image" <- w1491
        n587 = call <vilib>:"IMAQdx Configure Grab.vi"("error in"=w1493, "Number of Buffers"=u32 5, "Session In"=w1495) -> ("error out"=w1492:errorcluster, "Session Out"=w1490:T4)  [unwired: 7 in]
        n588 = Bundle By Name(cluster=w1499, "IMAQ"=w1491, "USBCam"=w1490) -> (w1497:T15)
        n589 = Merge Errors(w1501, w1492) -> (w1498:errorcluster)
        n590 = case shown="No Error" w1498 {
          tunnel: w1497 -> [w1509 w1510]
          tunnel: [w1507 w1510] -> w1496
          frame No Error {
            n591 = Bundle By Name(cluster=w1509, "Sys Status.USB Cam"=TRUE) -> (w1507:T15)
            n592 = property on="Preview" class="Bool (strict)"("DisabledEnum"=T6."Enabled" ("Disabled")) -> ()  [unwired: 2 in, 2 out]
          }
          frame Error {
          }
        }
        n593 = call <vilib>:"Add State(s) to Queue__JKI_lib_State_Machine.vi"("State(s) in (\"\")"=w1505) -> ("States Out"=w1504:string)  [unwired: 14 in]
      }
      frame "USBCam: Grab" {
        # "Template Separator\n(You can make a copy of, or modify, this frame)"
        n594 = Unbundle By Name(w1513) -> ("IMAQ"=w1517:T5, "USBCam"=w1518:T4)
        n595 = call <vilib>:"IMAQdx Get Image2.vi"("Buffer Number Mode (Next)"=IMAQdx_Buffer_Number_Mode."Last New", "error in"=w1515, "Image In"=w1517, "Session In"=w1518) -> ("error out"=w1516:errorcluster, "Image Out"=w1512:T5)  [unwired: 4 in, 2 out]
        n596 = local write "Image"(w1512) -> ()
        n597 = call <vilib>:"Add State(s) to Queue__JKI_lib_State_Machine.vi"("State(s) in (\"\")"=w1520) -> ("States Out"=w1519:string)  [unwired: 14 in]
      }
      frame "USBCam: Close" {
        # "Close USB camra\n(You can make a copy of, or modify, this frame)"
        n598 = Unbundle By Name(w1523) -> ("IMAQ"=w1525:T5, "USBCam"=w1528:T4, "Sys Status.USB Cam"=w1521:bool)
        n599 = case shown="True" w1521 {
          tunnel: w1528 -> [_ w1540]
          tunnel: [w1532 w1538] -> w1527
          tunnel: w1526 -> [w1532 w1537]
          tunnel: w1525 -> [_ w1536]
          tunnel: w1523 -> [w1531 w1535]
          tunnel: [w1531 w1534] -> w1524
          frame False {
          }
          frame True {
            n600 = call <vilib>:"IMAQdx Close Camera.vi"("error in"=w1537, "Session In"=w1540) -> ("error out"=w1539:errorcluster)  [unwired: 9 out]
            n601 = call "Imaq Dispose"("Image"=w1536, "error in (no error)"=w1539) -> ("error out"=w1538:errorcluster)  [unwired: 4 in]
            n602 = Bundle By Name(cluster=w1535, "Sys Status.USB Cam"=FALSE) -> (w1534:T15)
          }
        }
        n603 = call <vilib>:"Add State(s) to Queue__JKI_lib_State_Machine.vi"("State(s) in (\"\")"=w1530) -> ("States Out"=w1529:string)  [unwired: 14 in]
      }
      frame "---------- Dialog ----------" {
        # "Template Separator\n(You can make a copy of, or modify, this frame)"
        n604 = call <vilib>:"Add State(s) to Queue__JKI_lib_State_Machine.vi"("State(s) in (\"\")"=w1545) -> ("States Out"=w1544:string)  [unwired: 14 in]
      }
      frame "Dialog: DataSaved" {
        # "Show data saved dialog\n(You can make a copy of, or modify, this frame)"
        n605 = Unbundle By Name(w1550) -> ("SaveFilePath"=w1549:path)
        n606 = Path To String(path=w1549) -> (string=w1547:string)
        n607 = Concatenate Strings("Data successfully save at " ("message"), w1547) -> (w1546:string)
        n608 = One Button Dialog(message=w1546) -> ()  [unwired: 1 in, 1 out]
        n609 = call <vilib>:"Add State(s) to Queue__JKI_lib_State_Machine.vi"("State(s) in (\"\")"=w1554) -> ("States Out"=w1553:string)  [unwired: 14 in]
      }
      frame "---------- New Category ----------" {
        # "Template Separator\n(You can make a copy of, or modify, this frame)"
        n610 = call <vilib>:"Add State(s) to Queue__JKI_lib_State_Machine.vi"("State(s) in (\"\")"=w1559) -> ("States Out"=w1558:string)  [unwired: 14 in]
      }
      frame "New Category: 1" {
        # "Your code here.\n(You can make a copy of, or modify, this frame)"
        n611 = call <vilib>:"Add State(s) to Queue__JKI_lib_State_Machine.vi"("State(s) in (\"\")"=w1564) -> ("States Out"=w1563:string)  [unwired: 14 in]
      }
      frame "New Category: 2" {
        # "Your code here.\n(You can make a copy of, or modify, this frame)"
        n612 = call <vilib>:"Add State(s) to Queue__JKI_lib_State_Machine.vi"("State(s) in (\"\")"=w1569) -> ("States Out"=w1568:string)  [unwired: 14 in]
      }
    }
  }
  n613 = while {
    tunnel: w26 -> [w1574]
    tunnel: [w1571] -> w25
    tunnel: w8 -> [w1570]
    stop <- w1572 stop-if-true
    # "Scan loop (both pre and follow)"
    n614 = event shown="[1] <3D profile scan pts>: User Event" {
      selector: w1574 -> [_ _ _]
      dyn-events: [_ _ _] -> w1571
      timeout: 10 -> [_ _ _]
      tunnel: [_ _ TRUE] -> w1572
      tunnel: w1570 -> [_ w1576 _]
      event Timeout {
        n615 = event-data() -> ()  [unwired: 1 in, 3 out]
      }
      event User Event {
        w1586 = "\r"
        n616 = event-data() -> ("3D profile scan pts"=w1579:cluster{"x(mm)":dbl, "y(mm)":dbl, "z(mm)":dbl}[])  [unwired: 1 in, 4 out]
        n617 = flat-sequence {
          tunnel: w1579 -> [w1592]
          tunnel: [w1592] -> w1578
          frame #0 {
            n618 = local write "Poll grbl position?"(FALSE ("Poll position")) -> ()
            n619 = Wait (ms)(milliseconds to wait=u32 100) -> ()  [unwired: 1 out]
          }
        }
        n620 = for {
          shift-right: [w1596] -> w1581
          shift-left: errorcluster {"status"=FALSE, "code"=0, "source"=""} ("error out") -> [w1602]
          tunnel: w1578 -> [w1600] mode=indexing
          stop <- w1594 stop-if-true
          n621 = Unbundle By Name(w1600) -> ("x(mm)"=w1599:dbl, "y(mm)"=w1598:dbl, "z(mm)"=w1597:dbl)
          n622 = local read "AbortFlag"() -> (w1595:bool)
          n623 = Not A Number/Path/Refnum?(number/path/refnum=w1597) -> (NaN/Path/Refnum?=w1601:bool)
          n624 = case shown="False" w1601 {
            tunnel: w1602 -> [w1607 w1609]
            tunnel: [w1606 w1609] -> w1596
            tunnel: w1599 -> [w1605 _]
            tunnel: w1598 -> [w1604 _]
            tunnel: w1597 -> [w1603 _]
            frame False {
              # "if z not NaN, send"
              n625 = call "Go to Position.vi"("X (mm)"=w1605, "Y (mm)"=w1604, "Z (mm)"=w1603, "Wait for finish? (T)"=FALSE, "error in (no error)"=w1607) -> ("error out"=w1606:errorcluster)  [unwired: 10 in]
            }
            frame True {
              # "if z is NaN, do nothing"
            }
          }
          n626 = Or(x=w1596, y=w1595) -> (x .or. y?=w1594:bool)
        }
        n627 = while {
          shift-right: [w1618] -> w1577
          shift-left: w1581 -> [w1619]
          i -> [w1613]
          stop <- w1610 stop-if-true
          n628 = Greater?(x=w1613, y=500) -> (0:w1611:bool)
          n629 = call "Get Status.vi"("error in (no error)"=w1619) -> ("Status"=w1617:T9, "error out"=w1618:errorcluster)  [unwired: 10 in, 3 out]
          n630 = Wait (ms)(milliseconds to wait=u32 100) -> ()  [unwired: 1 out]
          n631 = Equal?(x=Status."Idle" ("Status"), y=w1617) -> (x = y?=w1614:bool)
          n632 = Or(x=w1614, y=w1611) -> (x .or. y?=w1610:bool)
        }
        n633 = Generate User Event(user event=w1576, event data cluster=TRUE ("event data"), error in=w1577) -> ()  [unwired: 1 in, 2 out]
        n634 = Concatenate Strings("$120=500" ("string"), w1586) -> (w1585:string)
        n635 = Concatenate Strings("$121=200" ("string"), w1586) -> (w1584:string)
        n636 = Concatenate Strings("$122=500" ("string"), w1586) -> (w1583:string)
        n637 = flat-sequence {
          tunnel: w1577 -> [_]
          frame #0 {
            n638 = local write "Poll grbl position?"(TRUE ("Poll position")) -> ()
          }
        }
        n639 = Build Array(w1585, w1584, w1583) -> (w1582:string[])
        n640 = for {
          tunnel: w1577 -> [w1621]
          tunnel: w1582 -> [w1620] mode=indexing
          n641 = call "Send-Receive Serial Port.vi"("Data to write"=w1620, "error in (no error)"=w1621) -> ()  [unwired: 12 in, 2 out]
        }
      }
      event User Event {
        n642 = event-data() -> ()  [unwired: 1 in, 5 out]
      }
    }
  }
  n643 = while {
    tunnel: w46 -> [w1626]
    tunnel: [w1625] -> w44
    tunnel: w38 -> [w1624]
    stop <- w1623 stop-if-true
    # "3D profile data aquisition loop"
    n644 = event shown="[1] <Start Range Finder>: User Event" {
      selector: w1626 -> [_ _]
      dyn-events: [_ _] -> w1625
      timeout: 5 -> [_ _]
      tunnel: w1624 -> [w1629 w1635]
      tunnel: [w1628 w1631] -> w1623
      event Timeout {
        n645 = event-data() -> ()  [unwired: 1 in, 3 out]
        n646 = Get Queue Status(queue=w1629) -> (error out=w1628:errorcluster)  [unwired: 2 in, 7 out]
      }
      event User Event {
        n647 = event-data() -> ()  [unwired: 1 in, 1 out]
        n648 = local read "Range Finder COM"() -> (w1637:refnum<visa-resource-name>)
        n649 = call "LabJack_FGV_T4.vi"("Operation(Read)"=enum16{"Write", "Read"}."Read" ("Operation")) -> ("error out"=w1633:errorcluster, "Read data"=w1632:i32)  [unwired: 9 in]
        n650 = while {
          tunnel: w1637 -> [w1663]
          shift-right: [w1657] -> w1631
          shift-left: errorcluster {"status"=FALSE, "code"=0, "source"=""} ("error in (no error)") -> [w1645]
          tunnel: w1635 -> [w1654]
          tunnel: w1633 -> [w1647]
          tunnel: w1632 -> [w1648]
          shift-right: [w1643] -> _
          shift-left: 0.0 ("relative seconds") -> [w1642]
          i -> [w1641]
          stop <- w1660 stop-if-true
          # "3D profile aquisition loop"
          n651 = VISA Read(VISA resource name=w1663, byte count=4, error in (no error)=w1645) -> (read buffer=w1651:string, error out=w1644:errorcluster)  [unwired: 2 out]
          "read buffer" <- w1651
          n652 = Quotient & Remainder(x=w1641, y=10) -> (x-y*floor(x/y)=w1639:i32)  [unwired: 1 out]
          n653 = String Length(string=w1651) -> (length=w1661:i32)
          n654 = call "LJM_eReadName.vi"("Handle In"=w1648, "Name"="DIO4_EF_READ_A_F", "error in"=w1647) -> ("Value"=w1656:dbl, "error out"=w1646:errorcluster)  [unwired: 10 in, 1 out]
          "X encoder count" <- w1656
          n655 = Equal To 0?(x=w1639) -> (x = 0?=w1638:bool)
          n656 = Equal?(x=w1661, y=3) -> (x = y?=w1649:bool)
          n657 = call <vilib>:"High Resolution Relative Seconds.vi"() -> ("relative seconds"=w1643:dbl)
          n658 = Multiply(x=w1656, y=0.0025) -> (x*y=w1653:dbl)
          "X (mm)" <- w1653
          n659 = case shown="True" w1638 {
            tunnel: w1643 -> [_ w1668]
            tunnel: w1642 -> [_ w1667]
            frame False {
            }
            frame True {
              n660 = Subtract(x=w1668, y=w1667) -> (x-y=w1666:dbl)
              n661 = Multiply(x=w1666, y=1000.0) -> (x*y=→"dt polling (ms)":dbl)
            }
          }
          n662 = case shown="False" w1649 {
            tunnel: w1651 -> [_ w1676]
            tunnel: [0.0 ("Distance(mm)") w1675] -> w1650
            frame False {
            }
            frame True {
              n663 = call "BinaryToMilimeter.vi"("Hex string"=w1676) -> ("Distance(mm)"=w1675:dbl)  [unwired: 10 in]
            }
          }
          "Z Distance(mm)" <- w1650
          n664 = Merge Errors(w1644, w1646) -> (w1657:errorcluster)
          n665 = case shown="True" w1649 {
            tunnel: w1654 -> [_ w1673]
            tunnel: w1653 -> [_ w1671]
            tunnel: w1650 -> [_ w1670]
            frame False {
            }
            frame True {
              n666 = Bundle(w1671, 0.0, "Distance(mm)"=w1670) -> (w1672:cluster{dbl, dbl, "Distance(mm)":dbl})  [unwired: 1 in]
              n667 = Enqueue Element(queue=w1673, element=w1672) -> ()  [unwired: 2 in, 3 out]
            }
          }
          n668 = Or(x=w1657, y="AccuRangeLoopStopFlag") -> (x .or. y?=w1660:bool)
        }
        "3D scan" <- w1631
      }
    }
  }
  n669 = while {
    tunnel: w13 -> [w1680]
    stop <- w1678 stop-if-true
    # "Waveform display loop"
    n670 = Wait (ms)(milliseconds to wait=u32 20) -> ()  [unwired: 1 out]
    n671 = Wait on Notification(notifier=w1680) -> (notification=→"PPIX intensity trace":dbl, error out=w1678:errorcluster)  [unwired: 3 in, 2 out]
  }
  n672 = while {
    tunnel: w22 -> [w1685]
    tunnel: w13 -> [w1683]
    tunnel: [w1682] -> w17
    tunnel: w4 -> [w1681]
    stop <- w1684 stop-if-true
    # "FLIm DAQ"
    n673 = event shown="[0] <Start FLIm>: User Event" {
      selector: w1685 -> [_ _ _]
      dyn-events: [_ _ _] -> w1682
      timeout: 5 -> [_ _ _]
      tunnel: [FALSE FALSE TRUE] -> w1684
      tunnel: w1683 -> [w1696 _ _]
      tunnel: w1681 -> [w1694 _ _]
      event User Event {
        n674 = event-data() -> ("Time"=→"LocationPollingStart":u32)  [unwired: 1 in, 4 out]
        n675 = Flush Queue(queue=w1694) -> (queue out=w1689:refnum<queue>)  [unwired: 1 in, 2 out]
        n676 = call "LabJack_FGV_T4.vi"("Operation(Read)"=enum16{"Write", "Read"}."Read" ("Operation")) -> ("error out"=w1692:errorcluster, "Read data"=w1691:i32)  [unwired: 9 in]
        n677 = Tick Count (ms)() -> (millisecond timer value=w1688:u32)
        n678 = while {
          tunnel: w1696 -> [w1721]
          shift-right: [w1707] -> _
          shift-left: 0.0 ("relative seconds") -> [w1720]
          tunnel: w1689 -> [w1716]
          tunnel: w1692 -> [w1701]
          tunnel: w1691 -> [w1714]
          tunnel: w1688 -> [w1698]
          stop <- w1708 stop-if-true
          n679 = call <vilib>:"High Resolution Relative Seconds.vi"() -> ("relative seconds"=w1707:dbl)
          n680 = Subtract(x=w1707, y=w1720) -> (x-y=w1706:dbl)
          n681 = call <userlib>:"Tick Count (ms)__ogtk.vi"("error in (no error)"=w1701) -> ("error out"=w1700:errorcluster, "millisecond timer value"=w1699:u32)  [unwired: 9 in]
          n682 = Multiply(x=w1706, y=1000.0) -> (x*y=w1704:dbl)
          n683 = local write "dt polling (ms)"(w1704) -> ()
          n684 = Subtract(x=w1699, y=w1698) -> (x-y=w1697:u32)
          n685 = call "LJM_eReadName.vi"("Handle In"=w1714, "Name"="DIO4_EF_READ_A_F", "error in"=w1700) -> ("Value"=w1702:dbl, "error out"=w1718:errorcluster)  [unwired: 10 in, 1 out]
          n686 = local write "X encoder count"(w1702) -> ()
          n687 = Multiply(x=w1702, y=0.0025) -> (x*y=w1703:dbl)
          n688 = local write "X (mm)"(w1703) -> ()
          n689 = Send Notification(notification=w1697, notifier=w1721) -> (error out=w1719:errorcluster)  [unwired: 1 in, 1 out]
          n690 = Bundle(w1697, w1703) -> (w1713:cluster{u32, dbl})  [unwired: 1 in]
          n691 = Enqueue Element(queue=w1716, element=w1713) -> (error out=w1715:errorcluster)  [unwired: 2 in, 2 out]
          n692 = Merge Errors(w1719, w1718, w1715) -> (w1709:errorcluster)
          n693 = Not(x="FollowScan") -> (.not. x?=w1710:bool)
          n694 = Or(x=w1710, y=w1709) -> (x .or. y?=w1708:bool)
        }
      }
      event Timeout {
        n695 = event-data() -> ()  [unwired: 1 in, 3 out]
      }
      event User Event {
        n696 = event-data() -> ()  [unwired: 1 in, 5 out]
      }
    }
  }
  n697 = local write "Poll grbl position?"(TRUE) -> ()
  n698 = local write "Preview"(FALSE ("Preview")) -> ()
  n699 = property on="Preview" class="Bool (strict)"("DisabledEnum"=T6."Disabled and Grayed Out" ("Disabled")) -> ()  [unwired: 2 in, 2 out]
  n700 = Unregister For Events(event registration refnum=w17, error in=w9) -> (error out=w16:errorcluster)
  n701 = Release Notifier(notifier=w13, error in (no error)=w9) -> (error out=w20:errorcluster)  [unwired: 1 in, 2 out]
  n702 = Unregister For Events(event registration refnum=w10, error in=w9) -> (error out=w7:errorcluster)
  n703 = Unregister For Events(event registration refnum=w44, error in=w43) -> (error out=w45:errorcluster)
  n704 = Unregister For Events(event registration refnum=w25, error in=w9) -> (error out=w24:errorcluster)
  n705 = Destroy User Event(user event=w8, error in=w7) -> (error out=w2:errorcluster)
  n706 = Release Queue(queue=w38, error in (no error)=w9) -> (error out=w40:errorcluster)  [unwired: 1 in, 2 out]
  n707 = Destroy User Event(user event=w29, error in=w45) -> (error out=w33:errorcluster)
  n708 = Destroy User Event(user event=w19, error in=w24) -> (error out=w23:errorcluster)
  n709 = Destroy User Event(user event=w1, error in=w9) -> (error out=w14:errorcluster)
  n710 = Merge Errors(w2, w40, w33, w9, w23, w20, w18, w16, w14) -> (w39:errorcluster)
  n711 = call <vilib>:"Simple Error Handler.vi"("error in (no error)"=w39) -> ()  [unwired: 4 in, 5 out]
